vi "Run Process.vi"(0 "Time Left X":refnum<vi>, 1 "Completion X":refnum<vi>, 2 "Current Cycle Display X":refnum<vi>, 3 "ALD Sequence for Reactor X":refnum<vi>, 4 "Current Cycle Reactor X":refnum<vi>, 5 "Table Position Reactor X":refnum<vi>, 6 "Stop / Start Reactor X":refnum<vi>, 7 "System Idle X":refnum<vi>, 8 "Reactor Number (Base 0)":i32, 9 "Stop Program":refnum<vi>, 11 "System Queue":refnum<vi>, 12 "System Constants":T2, 13 "System JSON Queue":refnum<vi>, 14 "Reactor Selector":T1(ring), 15 "Current Locks":refnum<vi>, 17 "Current Valve State":refnum<vi>, 19 "Debug Mode":refnum<vi>, 20 "Wait Before Start (s) X":refnum<vi>, 21 "Timer Reactor X":refnum<vi>, 22 "Countdown X":refnum<vi>, 23 "Pressure (mTorr) X":refnum<vi>, 24 "Recorded Pressure X":refnum<vi>, 25 "Lock Reentrance Rate":refnum<vi>, 26 "Valve Close Delay":refnum<vi>) -> ()   [LabVIEW 2021]
uses:
  Valve State Machine.ctl
panel:
  out "Valves Per Shared Line":i32
  out "Number of Reactors":i32
  out "Valves Per Reactor":i32
  out "N2 Valves":i32[](array[numeric])
  out "Pump Valves":i32[](array[numeric])
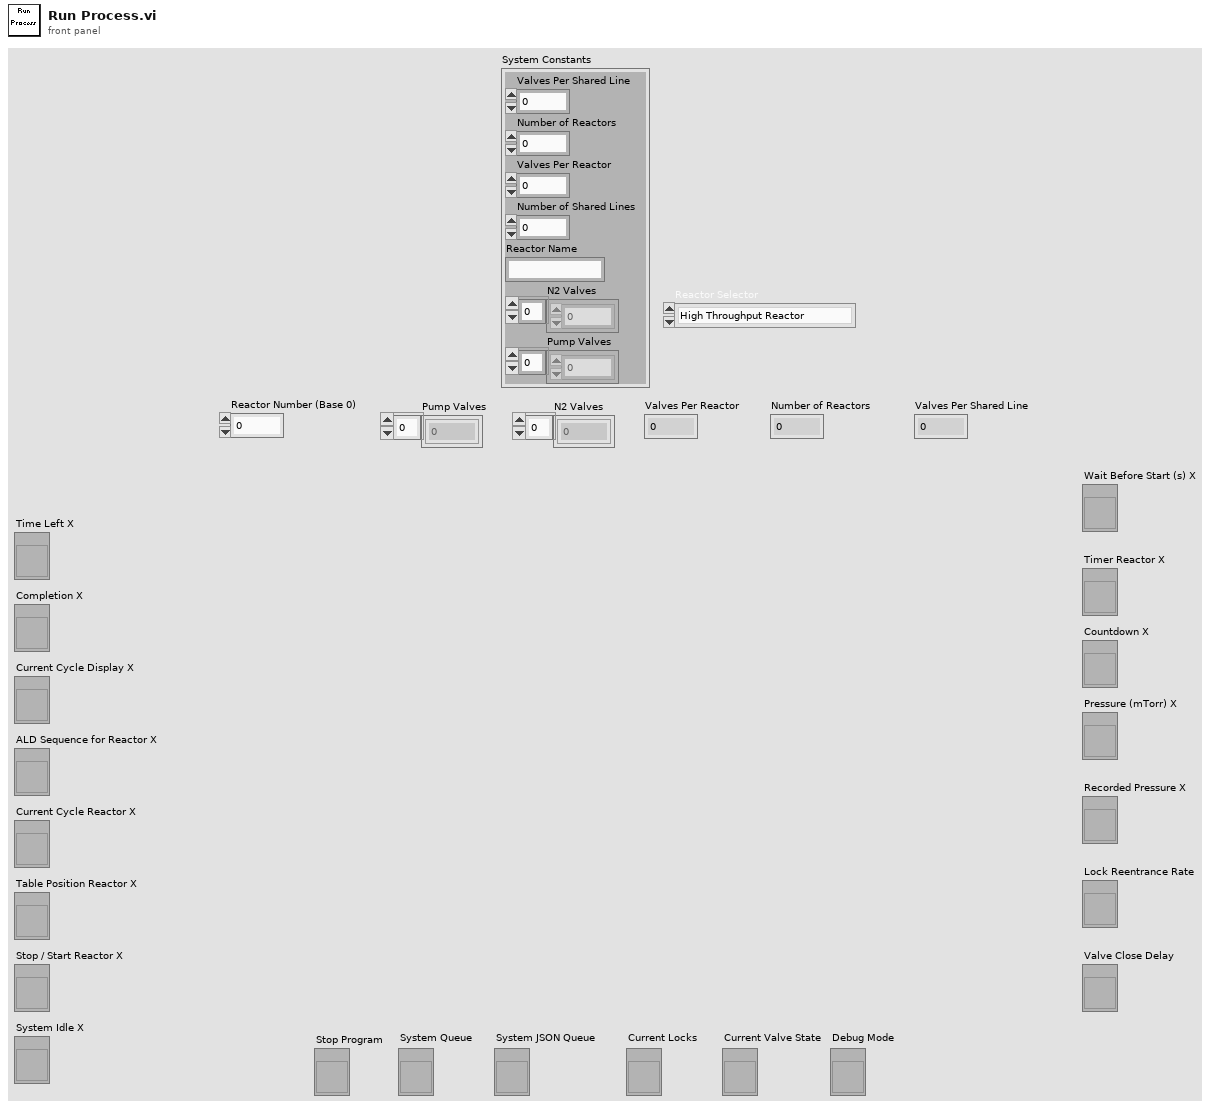
[diagram p1: front panel]
types:
  T1 = enum16{"High Throughput Reactor", "In Situ Reactor", "MLD Reactor"}
  T2 = cluster{"Valves Per Shared Line":i32, "Number of Reactors":i32, "Valves Per Reactor":i32, "Number of Shared Lines":i32, "Reactor Name":string, "N2 Valves":i32[], "Pump Valves":i32[]}
  T3 = typedef "Valve State Machine.ctl" = enum16{"0-Init Wait Before Start", "1-Wait Before Start", "2-Check Temp Request", "3-Claim Predose Pump Lock", "4-Init Predose Pump", "5-Wait Predose Pump", "6-Release Pump Lock", "7-Claim All Needed Locks", "8-Init N2Overlap", "9-Wait N2Overlap", "10-Init Pump Overlap", "11-Wait Pump Overlap", "12-Release Pump Lock", "13-Init Open Time", "14-Wait Open Time", "15-Release All Locks", "16-Init Hold", "17-Wait Hold", "18-Claim Pump Lock", "19-Init Pump Purge", "20-Wait Pump Purge", "21-Release Pump Lock", "22-Init Purge", "23-Wait Purge", "24-Check Purge Resume"}
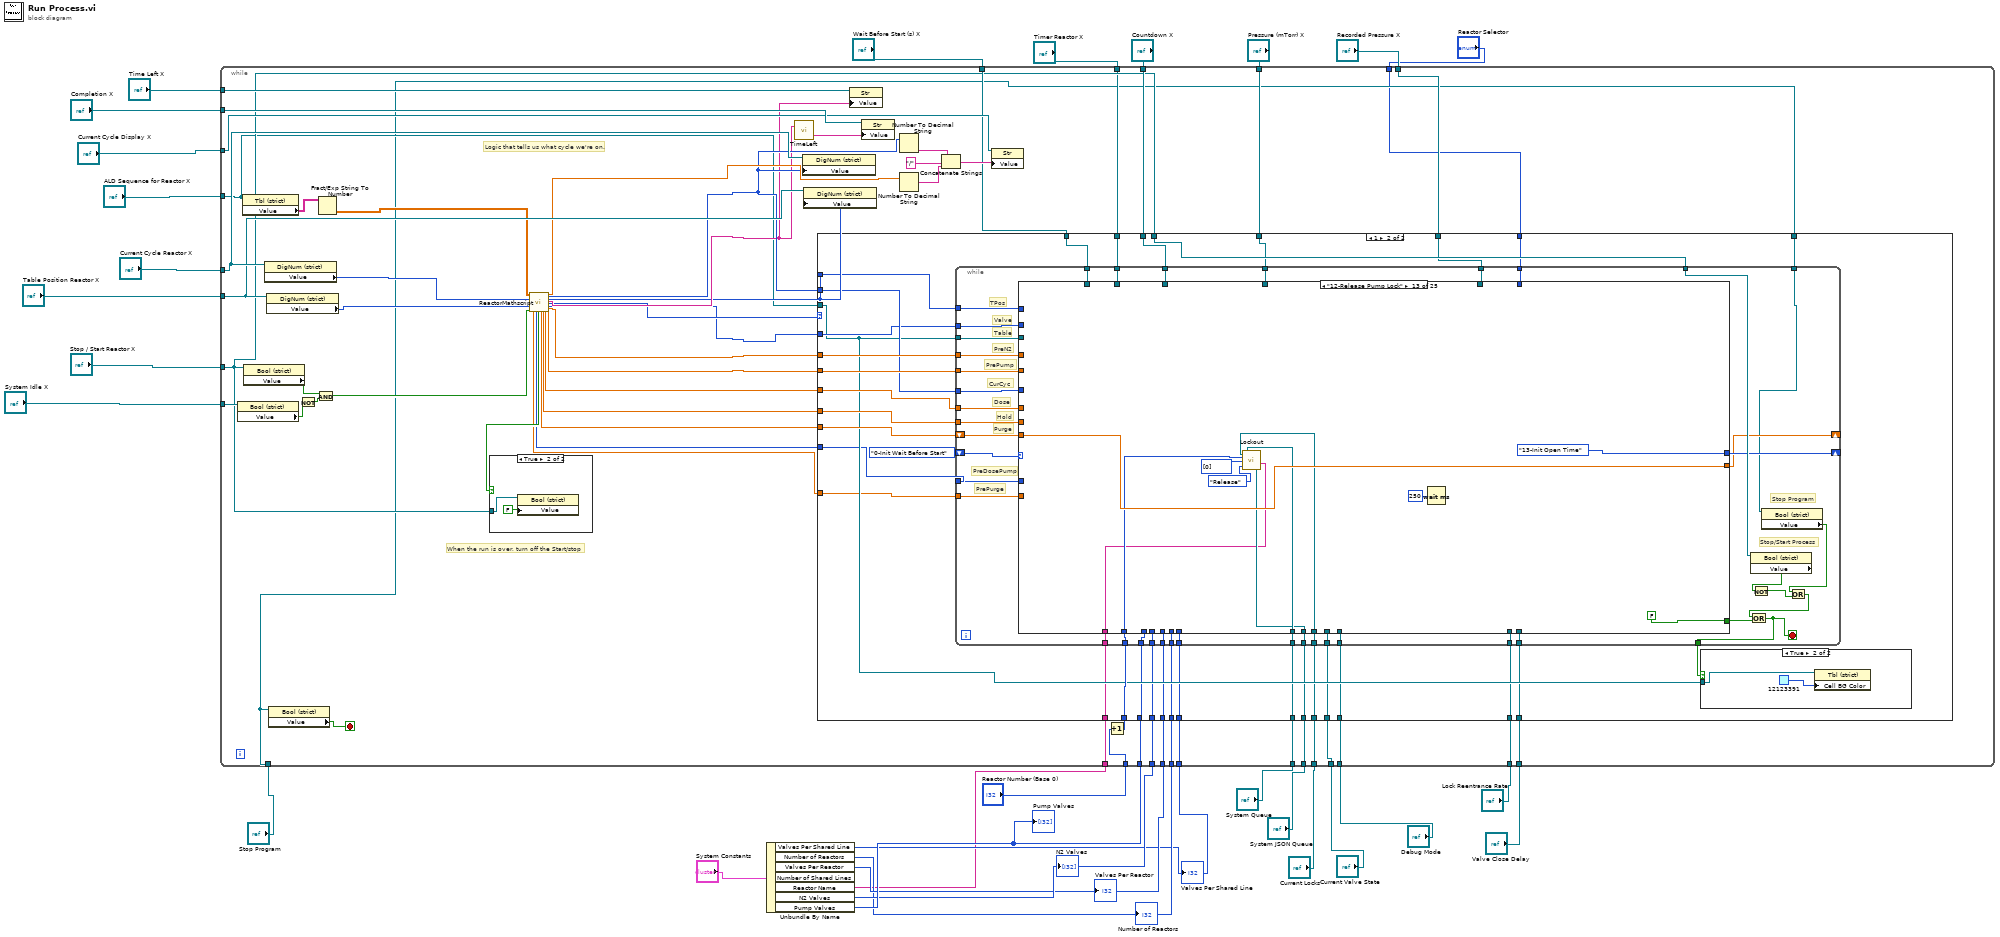
[diagram p0: block diagram]
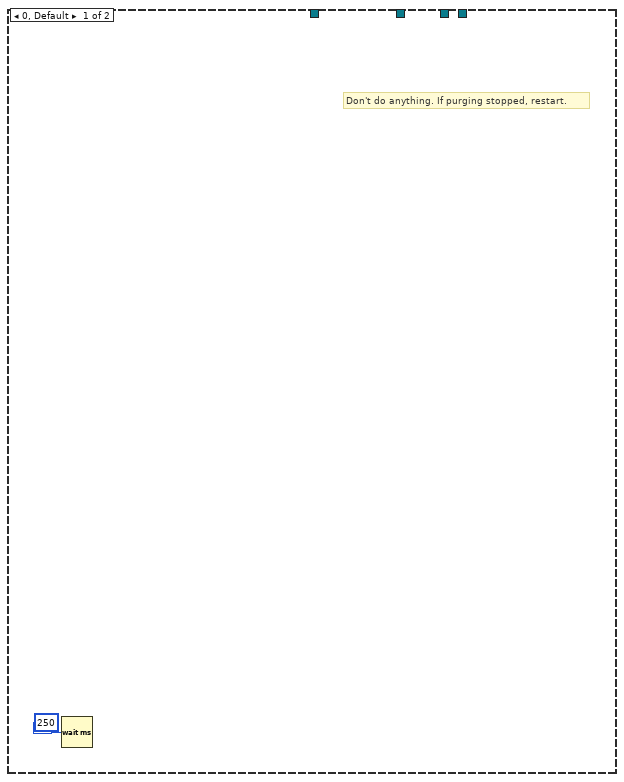
[diagram p3: hidden frame]
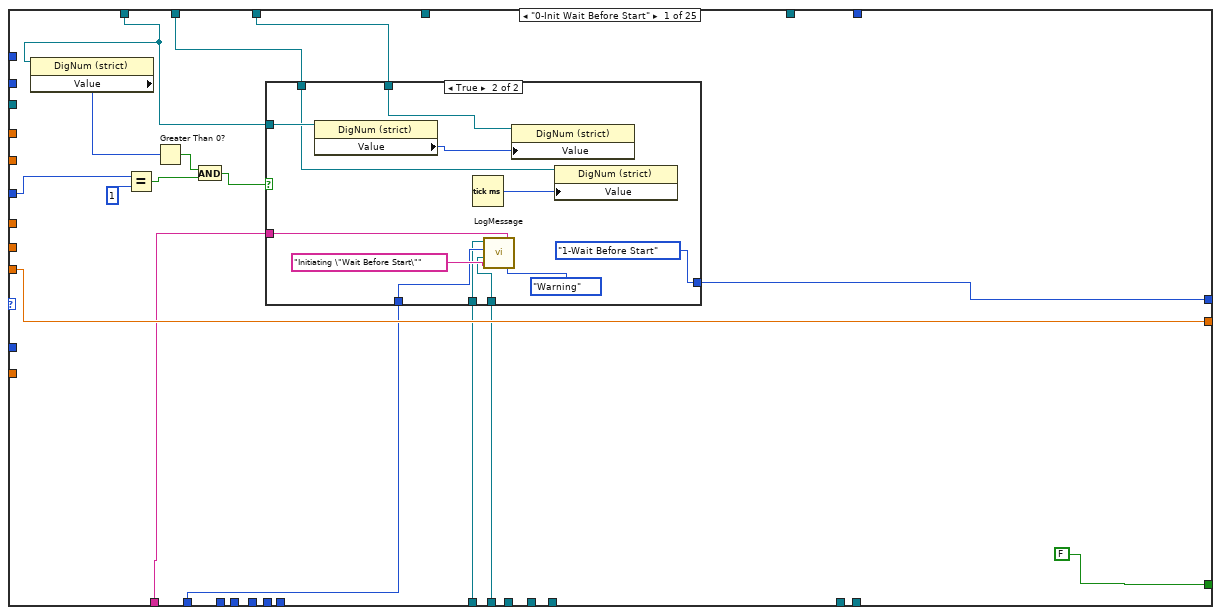
[diagram p5: hidden frame]
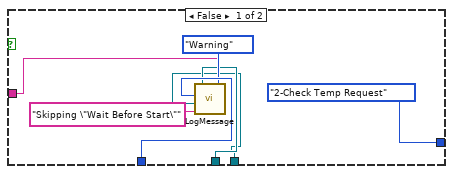
[diagram p6: hidden frame]
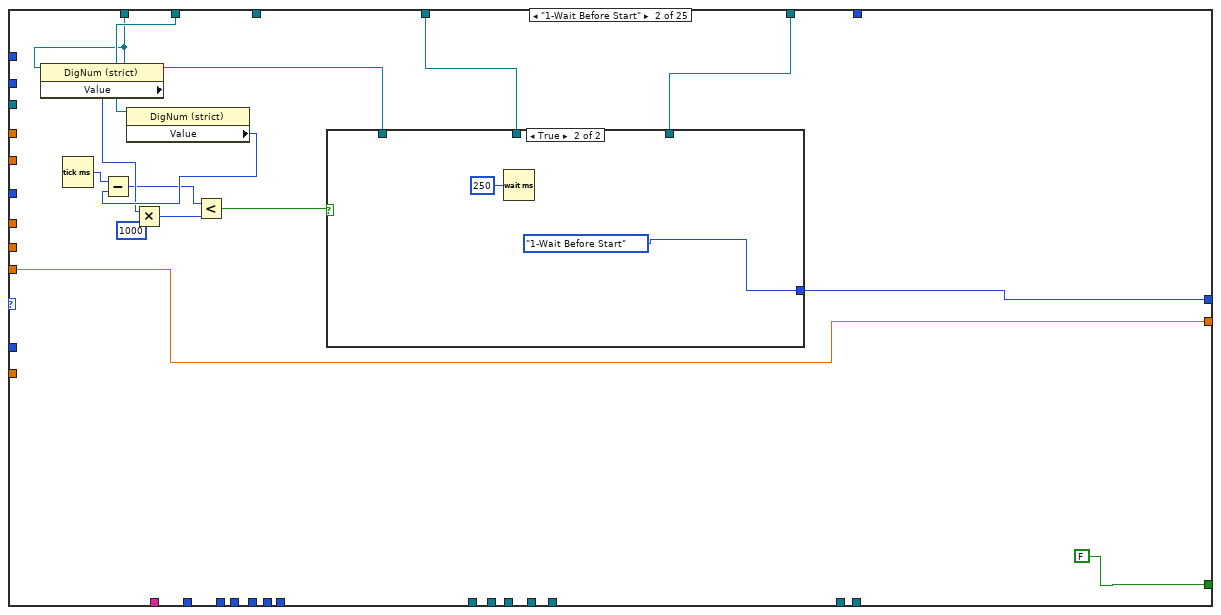
[diagram p7: hidden frame]
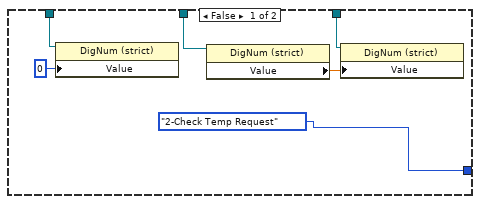
[diagram p8: hidden frame]
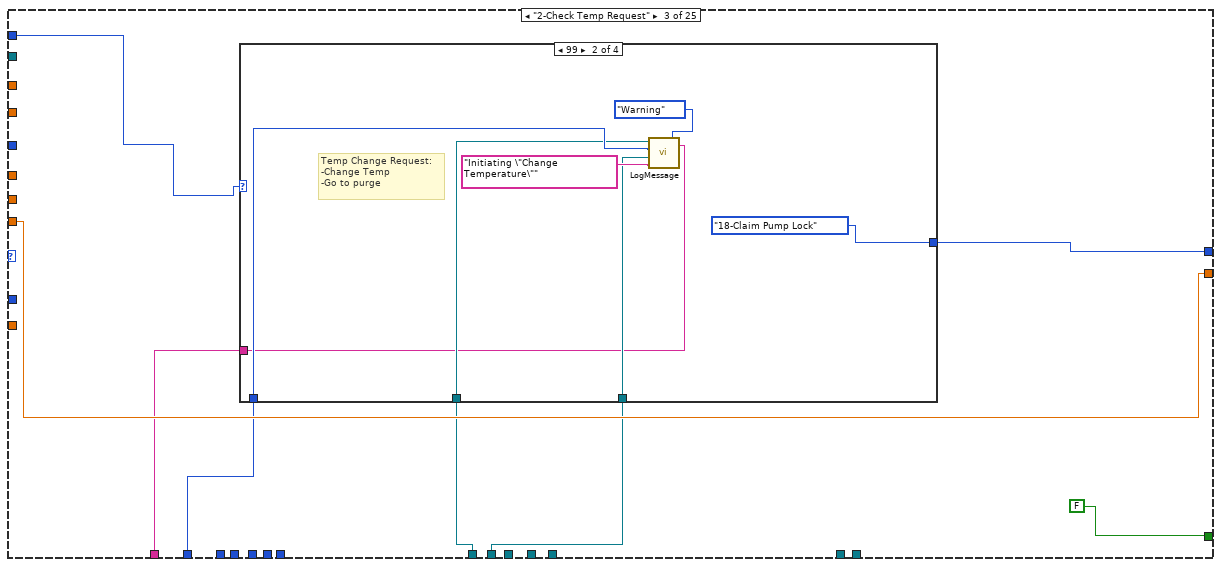
[diagram p9: hidden frame]
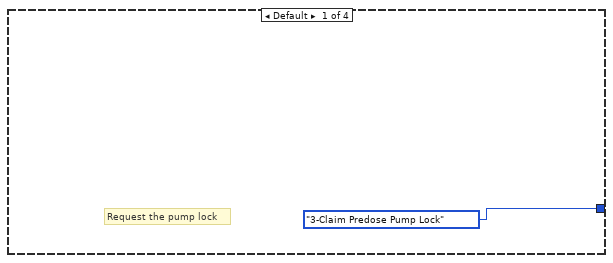
[diagram p10: hidden frame]
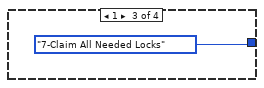
[diagram p11: hidden frame]
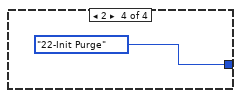
[diagram p12: hidden frame]
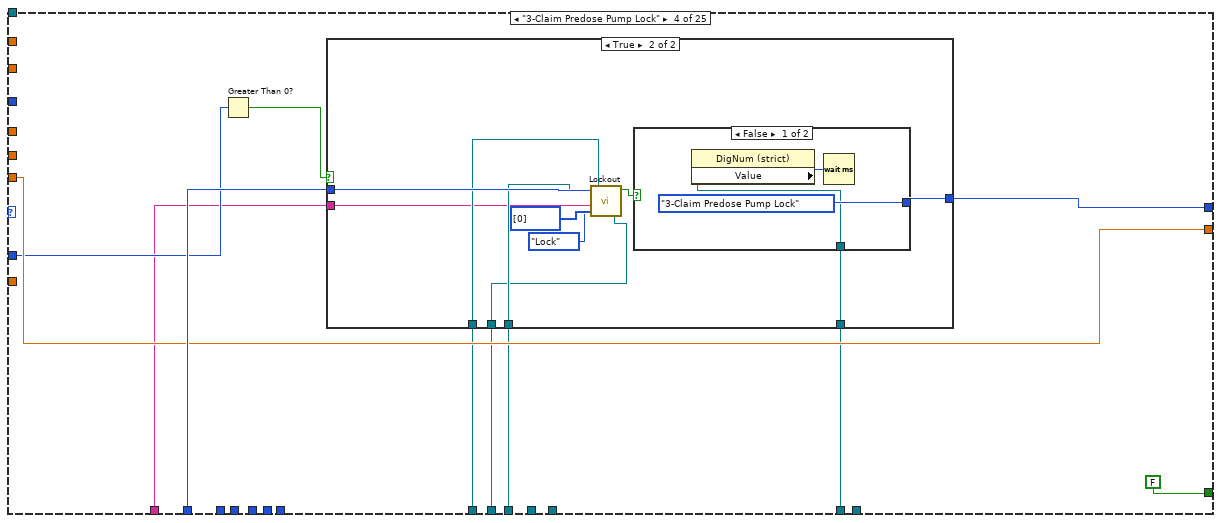
[diagram p13: hidden frame]
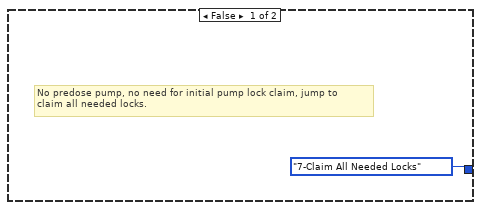
[diagram p14: hidden frame]
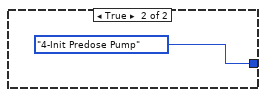
[diagram p15: hidden frame]
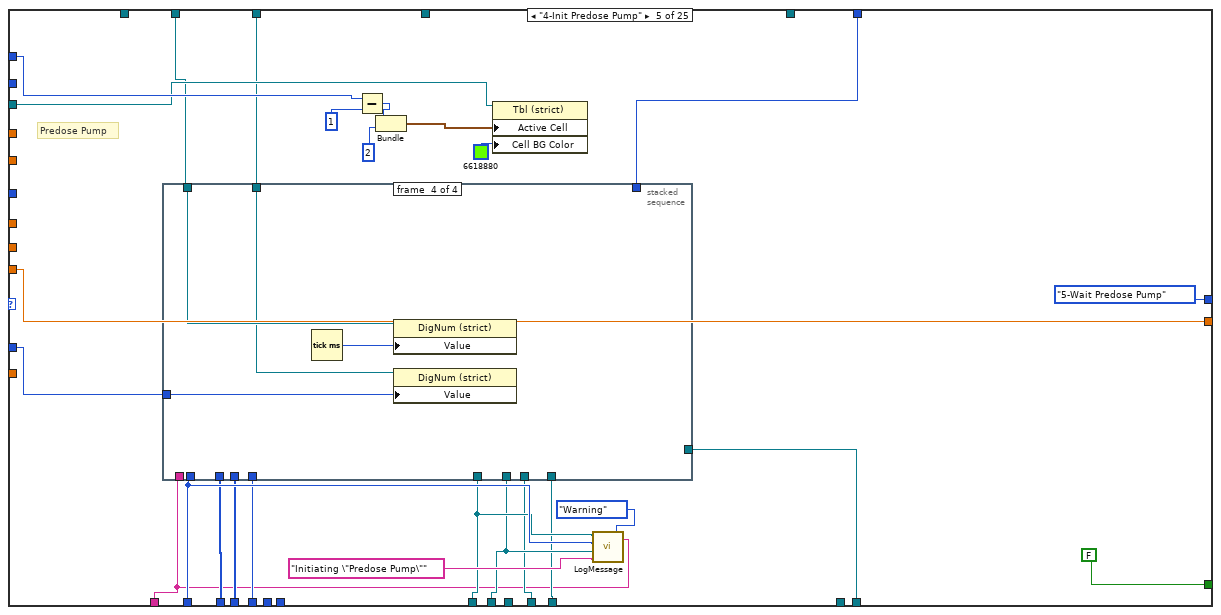
[diagram p16: hidden frame]
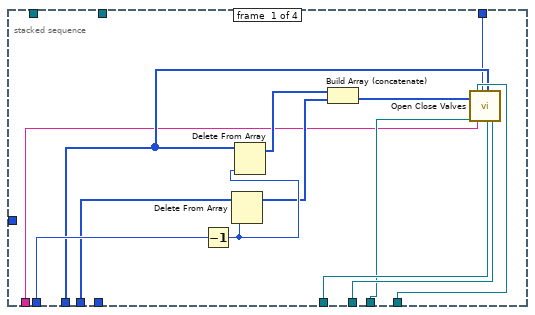
[diagram p17: hidden frame]
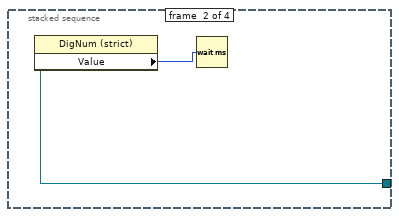
[diagram p18: hidden frame]
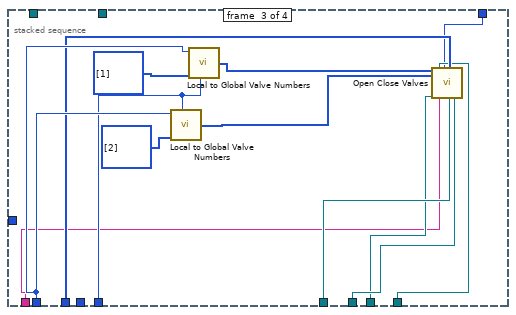
[diagram p19: hidden frame]
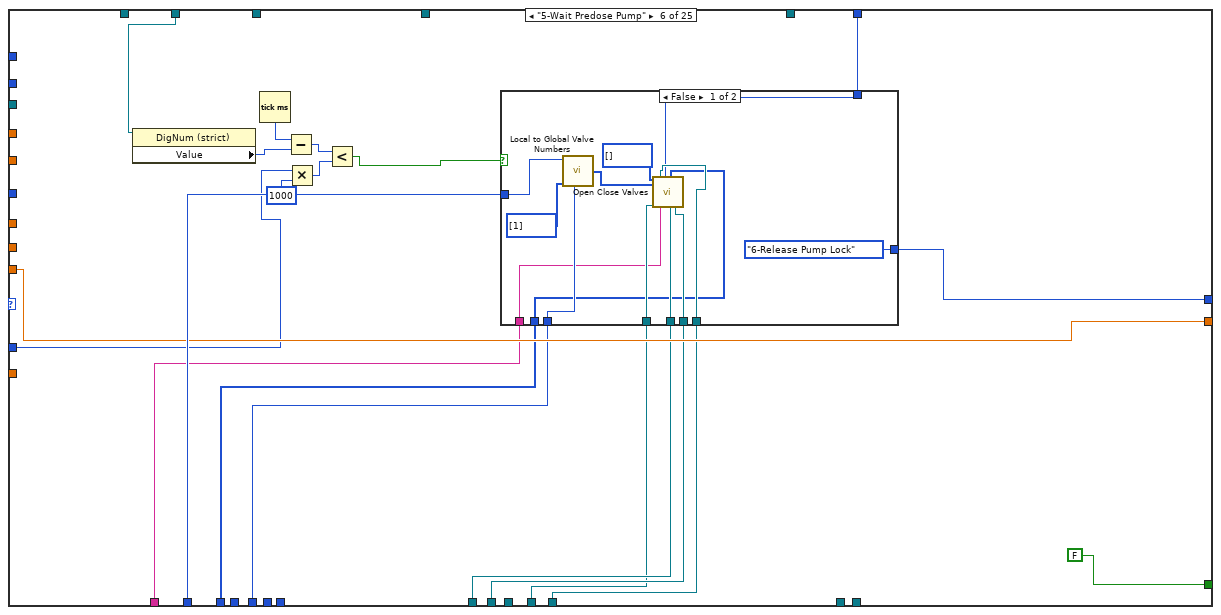
[diagram p20: hidden frame]
diagram:
  n1 = Unbundle By Name("System Constants") -> ("Valves Per Shared Line"=w3:i32, "Number of Reactors"=w4:i32, "Valves Per Reactor"=w5:i32, "Reactor Name"=w2:string, "N2 Valves"=w6:i32[], "Pump Valves"=w7:i32[])  [unwired: 1 out]
  "Pump Valves" <- w7
  "N2 Valves" <- w6
  "Valves Per Reactor" <- w5
  "Number of Reactors" <- w4
  "Valves Per Shared Line" <- w3
  n2 = while {
    tunnel: "Current Cycle Reactor X" -> [w85]
    tunnel: "Table Position Reactor X" -> [w81]
    tunnel: "ALD Sequence for Reactor X" -> [w49]
    tunnel: "System Idle X" -> [w88]
    tunnel: "Stop / Start Reactor X" -> [w60]
    tunnel: "Completion X" -> [w80]
    tunnel: "Time Left X" -> [w79]
    tunnel: "Current Cycle Display X" -> [w78]
    tunnel: "Wait Before Start (s) X" -> [w76]
    tunnel: "Countdown X" -> [w75]
    tunnel: "Pressure (mTorr) X" -> [w74]
    tunnel: "Recorded Pressure X" -> [w73]
    tunnel: "Reactor Number (Base 0)" -> [w72]
    tunnel: "Timer Reactor X" -> [w58]
    tunnel: "Stop Program" -> [w35]
    tunnel: "System Queue" -> [w45]
    tunnel: "System JSON Queue" -> [w44]
    tunnel: "Current Locks" -> [w43]
    tunnel: "Lock Reentrance Rate" -> [w42]
    tunnel: "Current Valve State" -> [w41]
    tunnel: "Debug Mode" -> [w40]
    tunnel: w7 -> [w39]
    tunnel: w6 -> [w38]
    tunnel: "Valve Close Delay" -> [w37]
    tunnel: w5 -> [w36]
    tunnel: w4 -> [w34]
    tunnel: w3 -> [w33]
    tunnel: w2 -> [w32]
    tunnel: "Reactor Selector" -> [w31]
    stop <- w46 stop-if-true
    # "When the run is over, turn off the Start/stop"
    # "Logic that tells us what cycle we're on."
    n3 = property class="Bool (strict)"(reference=w88) -> ("Value"=w86:bool)  [unwired: 1 in, 2 out]
    n4 = property class="Tbl (strict)"(reference=w49) -> ("Value"=w53:string[][])  [unwired: 1 in, 2 out]
    n5 = property class="Bool (strict)"(reference=w60) -> ("Value"=w87:bool)  [unwired: 1 in, 2 out]
    n6 = property class="DigNum (strict)"(reference=w85) -> ("Value"=w51:i32)  [unwired: 1 in, 2 out]
    n7 = property class="DigNum (strict)"(reference=w81) -> ("Value"=w52:i32)  [unwired: 1 in, 2 out]
    n8 = property class="Bool (strict)"(reference=w35) -> ("Value"=w46:bool)  [unwired: 1 in, 2 out]
    n9 = Not(x=w86) -> (.not. x?=w50:bool)
    n10 = And(x=w87, y=w50) -> (x .and. y?=w70:bool)
    n11 = Fract/Exp String To Number(string=w53) -> (number=w71:dbl[][])  [unwired: 3 in, 1 out]
    n12 = call "ReactorMathscript.vi"("T"=w71, "CurCycle"=w51, "TPos"=w52, "Run"=w70) -> ("PrePurge"=w47:dbl, "PreDosePump"=w48:i32, "StopRun"=w61:bool, "Purge"=w62:dbl, "Holds"=w63:dbl, "Dose"=w64:dbl, "TCyc"=w69:dbl, "CurCycle 2"=w68:i32, "TPos 2"=w56:i32, "TLeftStr"=w67:string, "Case"=w55:i32, "Valve"=w54:i32, "PreN2"=w66:dbl, "PrePump"=w65:dbl)  [unwired: 9 in, 1 out]
    n13 = case shown="True" w61 {
      tunnel: w60 -> [_ w90]
      frame False {
      }
      frame True {
        n14 = property class="Bool (strict)"(reference=w90, "Value"=FALSE) -> ()  [unwired: 1 in, 2 out]
      }
    }
    n15 = call "TimeLeft.vi"("Time Left"=w67) -> ("Completion"=w57:string)  [unwired: 2 in]
    n16 = property class="DigNum (strict)"(reference=w85, "Value"=w68) -> ()  [unwired: 1 in, 2 out]
    n17 = property class="DigNum (strict)"(reference=w81, "Value"=w56) -> ()  [unwired: 1 in, 2 out]
    n18 = property class="Str"(reference=w79, "Value"=w67) -> ()  [unwired: 1 in, 2 out]
    n19 = property class="Str"(reference=w80, "Value"=w57) -> ()  [unwired: 1 in, 2 out]
    n20 = Number To Decimal String(number=w68) -> (decimal integer string=w84:string)  [unwired: 1 in]
    n21 = Number To Decimal String(number=w69) -> (decimal integer string=w82:string)  [unwired: 1 in]
    n22 = Concatenate Strings(w84, "/", w82) -> (w77:string)
    n23 = property class="Str"(reference=w78, "Value"=w77) -> ()  [unwired: 1 in, 2 out]
    n24 = Increment(x=w72) -> (x+1=w59:i32)
    n25 = case shown="1" w55 {
      tunnel: w54 -> [_ w113]
      tunnel: w63 -> [_ w123]
      tunnel: w62 -> [_ w126]
      tunnel: w66 -> [_ w125]
      tunnel: w65 -> [_ w124]
      tunnel: w64 -> [_ w122]
      tunnel: w68 -> [_ w121]
      tunnel: w76 -> [_ w120]
      tunnel: w60 -> [_ w119]
      tunnel: w75 -> [_ w118]
      tunnel: w74 -> [_ w117]
      tunnel: w73 -> [_ w116]
      tunnel: w56 -> [_ w115]
      tunnel: w49 -> [_ w109]
      tunnel: w59 -> [_ w111]
      tunnel: w58 -> [_ w112]
      tunnel: w48 -> [_ w108]
      tunnel: w47 -> [_ w107]
      tunnel: w45 -> [_ w106]
      tunnel: w44 -> [_ w105]
      tunnel: w43 -> [_ w104]
      tunnel: w42 -> [_ w103]
      tunnel: w41 -> [_ w102]
      tunnel: w40 -> [_ w101]
      tunnel: w39 -> [_ w100]
      tunnel: w38 -> [_ w99]
      tunnel: w37 -> [_ w98]
      tunnel: w36 -> [_ w97]
      tunnel: w35 -> [_ w96]
      tunnel: w34 -> [_ w95]
      tunnel: w33 -> [_ w94]
      tunnel: w32 -> [_ w93]
      tunnel: w31 -> [_ w92]
      frame 0, Default {
        # "Don't do anything. If purging stopped, restart."
        n26 = Wait (ms)(milliseconds to wait=u32 250) -> ()  [unwired: 1 out]
      }
      frame 1 {
        n27 = while {
          shift-right: [w164] -> _
          shift-left: Valve_State_Machine."0-Init Wait Before Start" -> [w168]
          tunnel: w119 -> [w170]
          tunnel: w121 -> [w167]
          tunnel: w120 -> [w166]
          tunnel: w118 -> [w165]
          tunnel: w117 -> [w163]
          tunnel: w116 -> [w162]
          tunnel: w115 -> [w131]
          tunnel: w109 -> [w161]
          tunnel: w113 -> [w160]
          tunnel: w111 -> [w159]
          tunnel: w125 -> [w158]
          tunnel: w124 -> [w157]
          tunnel: w122 -> [w156]
          tunnel: w123 -> [w155]
          shift-right: [w153] -> _
          shift-left: w126 -> [w154]
          tunnel: w112 -> [w152]
          tunnel: [w150] -> w110
          tunnel: w108 -> [w149]
          tunnel: w107 -> [w148]
          tunnel: w106 -> [w147]
          tunnel: w105 -> [w146]
          tunnel: w104 -> [w145]
          tunnel: w103 -> [w144]
          tunnel: w102 -> [w143]
          tunnel: w101 -> [w142]
          tunnel: w100 -> [w141]
          tunnel: w99 -> [w140]
          tunnel: w98 -> [w139]
          tunnel: w97 -> [w138]
          tunnel: w96 -> [w136]
          tunnel: w95 -> [w133]
          tunnel: w94 -> [w132]
          tunnel: w93 -> [w130]
          tunnel: w92 -> [w129]
          stop <- w150 stop-if-true
          # "Stop/Start Process"
          # "Stop Program"
          # "PreDosePump"
          # "PrePurge"
          # "Purge"
          # "Hold"
          # "Dose"
          # "CurCyc"
          # "PrePump"
          # "PreN2"
          # "Table"
          # "Valve"
          # "TPos"
          n28 = case shown="\"12-Release Pump Lock\"" w168 {
            tunnel: [FALSE FALSE FALSE FALSE FALSE FALSE FALSE FALSE FALSE FALSE FALSE FALSE FALSE FALSE FALSE FALSE FALSE FALSE FALSE FALSE FALSE FALSE w1047 w1114 FALSE] -> w151
            tunnel: w167 -> [w176 _ _ _ _ _ _ _ _ _ _ _ _ _ _ _ _ _ _ _ _ _ _ _ _]
            tunnel: w166 -> [w180 w212 _ _ _ _ _ _ _ _ _ _ _ _ _ _ _ _ _ _ _ _ _ _ _]
            tunnel: w165 -> [w186 _ _ _ w283 _ _ _ w435 _ w606 _ _ w739 _ _ w862 _ _ w959 _ _ w1053 _ w1177]
            tunnel: [w182 w218 w234 w254 Valve_State_Machine."5-Wait Predose Pump" w349 Valve_State_Machine."7-Claim All Needed Locks" w397 w439 w543 w599 w688 Valve_State_Machine."13-Init Open Time" w734 w817 Valve_State_Machine."16-Init Hold" w857 w920 w935 w954 w1024 Valve_State_Machine."22-Init Purge" w1048 w1113 w1179] -> w164
            tunnel: w163 -> [_ w217 _ _ _ _ _ _ _ _ _ _ _ _ _ _ _ _ _ _ _ _ _ _ _]
            tunnel: w162 -> [_ w216 _ _ _ _ _ _ _ _ _ _ _ _ _ _ _ _ _ _ _ _ _ _ _]
            tunnel: w131 -> [_ _ _ _ w295 _ _ _ w434 _ w603 _ _ w738 _ _ w859 _ _ w956 _ _ w1051 _ _]
            tunnel: w161 -> [_ _ _ _ w294 _ _ _ w431 _ w604 _ _ w737 _ _ w860 _ _ w957 _ _ w1052 w1110 _]
            tunnel: w160 -> [_ _ w232 _ _ _ _ w375 w432 w532 w602 w676 _ w736 w805 _ w863 _ _ _ _ _ _ _ _]
            tunnel: w159 -> [w183 _ w231 w255 w285 w347 w371 w386 w433 w531 w601 w677 w715 w735 w806 w840 w858 _ w932 w955 _ w1033 w1050 w1111 _]
            tunnel: w158 -> [_ _ _ _ _ _ _ w393 w436 w533 _ _ _ _ _ _ _ _ _ _ _ _ _ _ _]
            tunnel: w157 -> [_ _ _ _ _ _ _ w389 _ _ w605 w679 _ _ _ _ _ _ _ _ _ _ _ _ _]
            tunnel: w156 -> [_ _ _ _ _ _ _ _ _ _ _ _ _ w740 w808 _ _ _ _ _ _ _ _ _ _]
            tunnel: w155 -> [_ _ _ _ _ _ _ _ _ _ _ _ _ _ _ _ w861 w910 _ _ _ _ _ _ _]
            tunnel: w154 -> [w184 w215 w233 w252 w288 w346 w372 w387 w430 w541 w598 w686 w717 w732 w815 w841 w855 w918 w933 w952 w1022 w1035 w1049 w1104 w1176]
            tunnel: [w184 w215 w233 w252 w288 w346 w372 w387 w430 w541 w598 w686 w717 w732 w815 w841 w855 w918 w933 w952 w1022 w1035 w1049 w1112 w1176] -> w153
            tunnel: w152 -> [w181 w214 _ _ w287 w339 _ _ w429 w534 w597 w678 _ w731 w807 _ w854 w911 _ w951 w1015 _ w1046 w1102 _]
            tunnel: w149 -> [_ _ _ w251 w282 w338 _ _ _ _ _ _ _ _ _ _ _ _ _ _ _ _ _ _ _]
            tunnel: w148 -> [_ _ _ _ _ _ _ _ _ _ _ _ _ _ _ _ _ _ _ w950 w1014 _ _ _ _]
            tunnel: w147 -> [w173 _ w230 w249 w281 w337 w367 w381 w426 w525 w591 w673 w712 w728 w798 w836 w848 _ w928 w945 _ w1030 w1044 w1099 w1169]
            tunnel: w146 -> [w172 _ w229 w248 w280 w336 w368 w382 w425 w524 w590 w672 w711 w727 w797 w835 w847 _ w927 w944 _ w1029 w1045 w1098 w1170]
            tunnel: w145 -> [_ _ _ w250 _ _ w366 w380 _ _ _ _ w710 _ _ w837 _ _ w926 _ _ w1031 _ _ w1171]
            tunnel: w144 -> [_ _ _ w247 _ _ _ w379 _ _ _ _ _ _ _ _ _ _ w925 _ _ _ _ _ w1168]
            tunnel: w143 -> [_ _ _ _ w279 w335 _ _ w422 w527 w589 w675 _ w729 w800 _ w849 _ _ w946 _ _ w1041 w1101 _]
            tunnel: w142 -> [_ _ _ _ w278 w334 _ _ w423 w526 w588 w674 _ w730 w799 _ w846 _ _ w943 _ _ w1042 _ _]
            tunnel: w141 -> [_ _ _ _ w277 w332 _ _ w421 w523 w593 w668 _ w722 w801 _ w850 _ _ w949 _ _ w1043 _ _]
            tunnel: w140 -> [_ _ _ _ w276 _ _ _ w420 _ w592 _ _ _ _ _ _ _ _ w948 _ _ _ _ _]
            tunnel: w139 -> [_ _ _ _ w275 _ _ _ w419 _ w587 _ _ w726 _ _ _ _ _ w942 _ _ _ _ _]
            tunnel: w138 -> [_ _ _ _ w274 w333 _ _ w427 w529 w595 w671 _ w724 w804 _ w853 _ _ w947 _ _ w1040 w1100 _]
            tunnel: w133 -> [_ _ _ _ _ _ _ _ w428 w530 w594 w670 _ w725 w803 _ w852 _ _ _ _ _ _ _ _]
            tunnel: w132 -> [_ _ _ _ _ _ _ _ w424 w528 w596 w669 _ w723 w802 _ w851 _ _ _ _ _ _ _ _]
            tunnel: w130 -> [w171 _ w228 w246 w273 w331 w365 w378 w418 w522 w586 w667 w709 w721 w796 w834 w845 _ w924 w941 _ w1028 w1039 w1097 w1167]
            tunnel: w129 -> [_ _ _ _ w272 w330 _ _ w417 w521 w585 w666 _ w720 w795 _ w844 _ _ w940 _ _ w1038 _ _]
            frame "0-Init Wait Before Start" {
              n29 = property class="DigNum (strict)"(reference=w180) -> ("Value"=w179:i32)  [unwired: 1 in, 2 out]
              n30 = Equal?(x=w176, y=1) -> (x = y?=w174:bool)
              n31 = Greater Than 0?(x=w179) -> (x > 0?=w178:bool)
              n32 = And(x=w178, y=w174) -> (x .and. y?=w177:bool)
              n33 = case shown="True" w177 {
                tunnel: w180 -> [_ w205]
                tunnel: w186 -> [_ w204]
                tunnel: w183 -> [w191 w198]
                tunnel: [Valve_State_Machine."2-Check Temp Request" Valve_State_Machine."1-Wait Before Start"] -> w182
                tunnel: w181 -> [_ w201]
                tunnel: w173 -> [w189 w196]
                tunnel: w172 -> [w188 w195]
                tunnel: w171 -> [w187 w194]
                frame False {
                  n34 = call "LogMessage.vi"("Type"=enum16{"Locks", "Warning"}."Warning", "Reactor Name"=w187, "Log Entry"="Skipping \"Wait Before Start\"", "System JSON Queue"=w188, "ID Number"=w191, "System Queue"=w189) -> ()
                }
                frame True {
                  n35 = property class="DigNum (strict)"(reference=w205) -> ("Value"=w203:i32)  [unwired: 1 in, 2 out]
                  n36 = Tick Count (ms)() -> (millisecond timer value=w200:u32)
                  n37 = call "LogMessage.vi"("Type"=enum16{"Locks", "Warning"}."Warning", "Reactor Name"=w194, "Log Entry"="Initiating \"Wait Before Start\"", "System JSON Queue"=w195, "ID Number"=w198, "System Queue"=w196) -> ()
                  n38 = property class="DigNum (strict)"(reference=w204, "Value"=w203) -> ()  [unwired: 1 in, 2 out]
                  n39 = property class="DigNum (strict)"(reference=w201, "Value"=w200) -> ()  [unwired: 1 in, 2 out]
                }
              }
            }
            frame "1-Wait Before Start" {
              n40 = property class="DigNum (strict)"(reference=w212) -> ("Value"=w209:i32)  [unwired: 1 in, 2 out]
              n41 = Tick Count (ms)() -> (millisecond timer value=w213:u32)
              n42 = property class="DigNum (strict)"(reference=w214) -> ("Value"=w211:i32)  [unwired: 1 in, 2 out]
              n43 = Subtract(x=w213, y=w211) -> (x-y=w207:u32)
              n44 = Multiply(x=w209, y=1000) -> (x*y=w206:i32)
              n45 = Less?(x=w207, y=w206) -> (x < y?=w210:bool)
              n46 = case shown="True" w210 {
                tunnel: [Valve_State_Machine."2-Check Temp Request" Valve_State_Machine."1-Wait Before Start"] -> w218
                tunnel: w212 -> [w225 _]
                tunnel: w217 -> [w223 _]
                tunnel: w216 -> [w222 _]
                frame False {
                  n47 = property class="DigNum (strict)"(reference=w225, "Value"=0) -> ()  [unwired: 1 in, 2 out]
                  n48 = property class="DigNum (strict)"(reference=w223) -> ("Value"=w221:dbl)  [unwired: 1 in, 2 out]
                  n49 = property class="DigNum (strict)"(reference=w222, "Value"=w221) -> ()  [unwired: 1 in, 2 out]
                }
                frame True {
                  n50 = Wait (ms)(milliseconds to wait=u32 250 ("millisecond multiple")) -> ()  [unwired: 1 out]
                }
              }
            }
            frame "2-Check Temp Request" {
              n51 = case shown="99" w232 {
                tunnel: [Valve_State_Machine."3-Claim Predose Pump Lock" Valve_State_Machine."18-Claim Pump Lock" Valve_State_Machine."7-Claim All Needed Locks" Valve_State_Machine."22-Init Purge"] -> w234
                tunnel: w231 -> [_ w241 _ _]
                tunnel: w230 -> [_ w239 _ _]
                tunnel: w229 -> [_ w238 _ _]
                tunnel: w228 -> [_ w237 _ _]
                frame Default {
                  # "Request the pump lock"
                }
                frame 99 {
                  # "Temp Change Request:\n-Change Temp\n-Go to purge"
                  n52 = call "LogMessage.vi"("Type"=enum16{"Locks", "Warning"}."Warning", "Reactor Name"=w237, "Log Entry"="Initiating \"Change Temperature\"", "System JSON Queue"=w238, "ID Number"=w241, "System Queue"=w239) -> ()
                }
                frame 1 {
                }
                frame 2 {
                }
              }
            }
            frame "3-Claim Predose Pump Lock" {
              n53 = Greater Than 0?(x=w251) -> (x > 0?=w256:bool)
              n54 = case shown="True" w256 {
                tunnel: w255 -> [_ w266]
                tunnel: [Valve_State_Machine."7-Claim All Needed Locks" w267] -> w254
                tunnel: w250 -> [_ w262]
                tunnel: w249 -> [_ w261]
                tunnel: w248 -> [_ w260]
                tunnel: w247 -> [_ w259]
                tunnel: w246 -> [_ w258]
                frame False {
                  # "No predose pump, no need for initial pump lock claim, jump to\nclaim all needed locks."
                }
                frame True {
                  n55 = call "Lockout.vi"("Locks"=w262, "ID"=w266, "Queue System"=w261, "Request Type"=enum16{"Lock", "Release", "Check"}."Lock", "Request Array"=i32[] [0], "Reactor Name"=w258, "JSON Queue"=w260) -> ("Response"=w263:bool)  [unwired: 1 out]
                  n56 = case shown="False" w263 {
                    tunnel: [Valve_State_Machine."3-Claim Predose Pump Lock" Valve_State_Machine."4-Init Predose Pump"] -> w267
                    tunnel: w259 -> [w268 _]
                    frame False {
                      n57 = property class="DigNum (strict)"(reference=w268) -> ("Value"=w269:i32)  [unwired: 1 in, 2 out]
                      n58 = Wait (ms)(milliseconds to wait=w269) -> ()  [unwired: 1 out]
                    }
                    frame True {
                    }
                  }
                }
              }
            }
            frame "4-Init Predose Pump" {
              # "Predose Pump"
              n59 = stacked-sequence {
                tunnel: w285 -> [w307 _ w323 _]
                tunnel: w287 -> [_ _ _ w328]
                tunnel: w283 -> [_ _ _ w327]
                tunnel: w282 -> [_ _ _ w326]
                tunnel: w281 -> [w305 _ w317 _]
                tunnel: w280 -> [w304 _ w316 _]
                tunnel: w279 -> [w303 _ w315 _]
                tunnel: w278 -> [w302 _ w318 _]
                tunnel: w277 -> [w301 _ w319 _]
                tunnel: w276 -> [w300 _ _ _]
                tunnel: w275 -> [_ w311 _ _]
                tunnel: w274 -> [_ _ w320 _]
                tunnel: w273 -> [w299 _ w314 _]
                tunnel: w272 -> [w298 _ w313 _]
                frame #0 {
                  n60 = Decrement(x=w307) -> (x-1=w310:i32)
                  n61 = Delete From Array(array=w300, index=w310) -> (array with subset deleted=w308:i32[])  [unwired: 1 in, 1 out]
                  n62 = Delete From Array(array=w301, index=w310) -> (array with subset deleted=w309:i32[])  [unwired: 1 in, 1 out]
                  n63 = Build Array (concatenate)(w309, w308) -> (w306:i32[])
                  n64 = call "Open Close Valves.vi"("Valves to Close"=w306, "Current Valve State"=w303, "Debug Mode"=w302, "Reactor Name"=w299, "Reactor Selector"=w298, "Pump Valves"=w301, "System Queue"=w305, "JSON Queue"=w304) -> ()  [unwired: 12 in]
                }
                frame #1 {
                  n65 = property class="DigNum (strict)"(reference=w311) -> ("Value"=w312:i32)  [unwired: 1 in, 2 out]
                  n66 = Wait (ms)(milliseconds to wait=w312) -> ()  [unwired: 1 out]
                }
                frame #2 {
                  n67 = call "Local to Global Valve Numbers.vi"("Reactor ID #"=w323, "List of Local Valves"=i32[] [2], "Valves Per Reactor"=w320) -> ("List of Global Valves"=w321:i32[])  [unwired: 2 in]
                  n68 = call "Local to Global Valve Numbers.vi"("Reactor ID #"=w323, "List of Local Valves"=i32[] [1] ("Valves to Open"), "Valves Per Reactor"=w320) -> ("List of Global Valves"=w322:i32[])  [unwired: 2 in]
                  n69 = call "Open Close Valves.vi"("Valves to Open"=w322, "Valves to Close"=w321, "Current Valve State"=w315, "Debug Mode"=w318, "Reactor Name"=w314, "Reactor Selector"=w313, "Pump Valves"=w319, "System Queue"=w317, "JSON Queue"=w316) -> ()  [unwired: 11 in]
                }
                frame #3 {
                  n70 = Tick Count (ms)() -> (millisecond timer value=w329:u32)
                  n71 = property class="DigNum (strict)"(reference=w328, "Value"=w329) -> ()  [unwired: 1 in, 2 out]
                  n72 = property class="DigNum (strict)"(reference=w327, "Value"=w326) -> ()  [unwired: 1 in, 2 out]
                }
              }
              n73 = Subtract(x=w295, y=1) -> (x-y=w293:i32)
              n74 = Bundle(w293, 2) -> (w292:cluster{i32, i32})  [unwired: 1 in]
              n75 = property class="Tbl (strict)"(reference=w294, "Active Cell"=w292, "Cell BG Color"=u32 6618880) -> ()  [unwired: 1 in, 2 out]
              n76 = call "LogMessage.vi"("Type"=enum16{"Locks", "Warning"}."Warning", "Reactor Name"=w273, "Log Entry"="Initiating \"Predose Pump\"", "System JSON Queue"=w280, "ID Number"=w285, "System Queue"=w281) -> ()
            }
            frame "5-Wait Predose Pump" {
              n77 = property class="DigNum (strict)"(reference=w339) -> ("Value"=w342:i32)  [unwired: 1 in, 2 out]
              n78 = Tick Count (ms)() -> (millisecond timer value=w341:u32)
              n79 = Subtract(x=w341, y=w342) -> (x-y=w343:u32)
              n80 = Multiply(x=w338, y=1000) -> (x*y=w344:i32)
              n81 = Less?(x=w343, y=w344) -> (x < y?=w340:bool)
              n82 = case shown="False" w340 {
                tunnel: [Valve_State_Machine."6-Release Pump Lock" Valve_State_Machine."5-Wait Predose Pump"] -> w349
                tunnel: w347 -> [w361 _]
                tunnel: w337 -> [w357 _]
                tunnel: w336 -> [w356 _]
                tunnel: w335 -> [w355 _]
                tunnel: w334 -> [w354 _]
                tunnel: w333 -> [w353 _]
                tunnel: w332 -> [w352 _]
                tunnel: w331 -> [w351 _]
                tunnel: w330 -> [w350 _]
                frame False {
                  n83 = call "Local to Global Valve Numbers.vi"("Reactor ID #"=w361, "List of Local Valves"=i32[] [1], "Valves Per Reactor"=w353) -> ("List of Global Valves"=w359:i32[])  [unwired: 2 in]
                  n84 = call "Open Close Valves.vi"("Valves to Open"=i32[] [], "Valves to Close"=w359, "Current Valve State"=w355, "Debug Mode"=w354, "Reactor Name"=w351, "Reactor Selector"=w350, "Pump Valves"=w352, "System Queue"=w357, "JSON Queue"=w356) -> ()  [unwired: 11 in]
                }
                frame True {
                  n85 = Wait (ms)(milliseconds to wait=u32 250 ("millisecond multiple")) -> ()  [unwired: 1 out]
                }
              }
            }
            frame "6-Release Pump Lock" {
              n86 = call "Lockout.vi"("Locks"=w366, "ID"=w371, "Queue System"=w367, "Request Type"=enum16{"Lock", "Release", "Check"}."Release", "Request Array"=i32[] [0], "Reactor Name"=w365, "JSON Queue"=w368) -> ()  [unwired: 2 out]
            }
            frame "7-Claim All Needed Locks" {
              n87 = Not Equal?(x=w375, y=2) -> (x != y?=w394:bool)
              n88 = Greater Than 0?(x=w393) -> (x > 0?=w392:bool)
              n89 = Greater Than 0?(x=w389) -> (x > 0?=w390:bool)
              n90 = And(x=w394, y=w392) -> (x .and. y?=w391:bool)
              n91 = Or(x=w391, y=w390) -> (x .or. y?=w388:bool)
              n92 = Greater?(x=w375, y=50) -> (0:w377:bool)
              n93 = case shown="True" w388 {
                tunnel: [i32[] [] i32[] [0]] -> w398
                frame False {
                  # "Purge only"
                }
                frame True {
                }
              }
              n94 = case shown="True" w377 {
                tunnel: w398 -> [w409 w413]
                tunnel: [w409 w412] -> w385
                tunnel: w375 -> [_ w411]
                frame False {
                }
                frame True {
                  n95 = Quotient & Remainder(x=w411, y=10) -> (floor(x/y)=w416:i32)  [unwired: 1 out]
                  n96 = Subtract(x=w416, y=4) -> (x-y=w410:i32)
                  n97 = Build Array (concatenate)(w413, w410) -> (w412:i32[])
                }
              }
              n98 = call "Lockout.vi"("Locks"=w380, "ID"=w386, "Queue System"=w381, "Request Type"=enum16{"Lock", "Release", "Check"}."Lock", "Request Array"=w385, "Reactor Name"=w378, "JSON Queue"=w382) -> ("Response"=w383:bool)  [unwired: 1 out]
              n99 = case shown="False" w383 {
                tunnel: [Valve_State_Machine."6-Release Pump Lock" w404] -> w397
                tunnel: w375 -> [_ w405]
                tunnel: w379 -> [w401 _]
                frame False {
                  n100 = property class="DigNum (strict)"(reference=w401) -> ("Value"=w402:i32)  [unwired: 1 in, 2 out]
                  n101 = Wait (ms)(milliseconds to wait=w402) -> ()  [unwired: 1 out]
                }
                frame True {
                  n102 = case shown="1" w405 {
                    tunnel: [Valve_State_Machine."8-Init N2Overlap" Valve_State_Machine."10-Init Pump Overlap" Valve_State_Machine."22-Init Purge"] -> w404
                    frame Default {
                    }
                    frame 1 {
                    }
                    frame 2 {
                    }
                  }
                }
              }
            }
            frame "8-Init N2Overlap" {
              # "Pump Open\nNitrogen Open"
              n103 = Greater Than 0?(x=w436) -> (x > 0?=w437:bool)
              n104 = case shown="True" w437 {
                tunnel: [Valve_State_Machine."10-Init Pump Overlap" Valve_State_Machine."9-Wait N2Overlap"] -> w439
                tunnel: w436 -> [_ w456]
                tunnel: w435 -> [_ w457]
                tunnel: w434 -> [_ w471]
                tunnel: w433 -> [_ w459]
                tunnel: w432 -> [_ w444]
                tunnel: w431 -> [_ w467]
                tunnel: w429 -> [_ w463]
                tunnel: w428 -> [_ w455]
                tunnel: w427 -> [_ w454]
                tunnel: w426 -> [_ w452]
                tunnel: w425 -> [_ w451]
                tunnel: w424 -> [_ w453]
                tunnel: w423 -> [_ w450]
                tunnel: w422 -> [_ w449]
                tunnel: w421 -> [_ w448]
                tunnel: w420 -> [_ w447]
                tunnel: w419 -> [_ w446]
                tunnel: w418 -> [_ w442]
                tunnel: w417 -> [_ w441]
                frame False {
                }
                frame True {
                  n105 = Greater?(x=w444, y=50) -> (0:w445:bool)
                  n106 = case shown="True" w445 {
                    tunnel: [w515 w518] -> w462
                    tunnel: w459 -> [w511 w519]
                    tunnel: w455 -> [w509 _]
                    tunnel: w454 -> [w508 w517]
                    tunnel: w453 -> [w503 _]
                    tunnel: w444 -> [w507 _]
                    frame True {
                      n107 = Quotient & Remainder(x=w507, y=10) -> (floor(x/y)=w506:i32)  [unwired: 1 out]
                      n108 = Subtract(x=w506, y=5) -> (x-y=w504:i32)
                      n109 = Multiply(x=w504, y=w503) -> (x*y=w502:i32)
                      n110 = call "Local to Global Valve Numbers.vi"("Reactor ID #"=w511, "List of Local Valves"=i32[] [1], "Valves Per Reactor"=w508) -> ("List of Global Valves"=w510:i32[])  [unwired: 2 in]
                      n111 = Multiply(x=w508, y=w509) -> (x*y=w514:i32)
                      n112 = Add(x=w514, y=w502) -> (x+y=w513:i32)
                      n113 = Increment(x=w513) -> (x+1=w516:i32)
                      n114 = Build Array (concatenate)(w510, w516) -> (w515:i32[])
                    }
                    frame False {
                      n115 = call "Local to Global Valve Numbers.vi"("Reactor ID #"=w519, "List of Local Valves"=i32[] [1, 2], "Valves Per Reactor"=w517) -> ("List of Global Valves"=w518:i32[])  [unwired: 2 in]
                    }
                  }
                  n116 = call "Convert Recipe Valve to Valve List.vi"("Valves on Shared Lines"=w453, "Valves Per Reactor"=w454, "Number of Reactors"=w455, "Reactor ID#"=w459, "Valve Number"=w444) -> ("Valve List"=w466:i32[])  [unwired: 10 in]
                  n117 = Build Array (concatenate)(w466, w462) -> (w465:i32[])
                  n118 = Subtract(x=w471, y=1) -> (x-y=w474:i32)
                  n119 = Bundle(w474, 3) -> (w470:cluster{i32, i32})  [unwired: 1 in]
                  n120 = Decrement(x=w459) -> (x-1=w461:i32)
                  n121 = property class="Tbl (strict)"(reference=w467, "Cell BG Color"=u32 12123391, "Active Cell"=w470, "Cell BG Color"=u32 16318208) -> ()  [unwired: 1 in, 2 out]
                  n122 = stacked-sequence {
                    tunnel: w465 -> [_ _ w496 _]
                    tunnel: w463 -> [_ _ _ w499]
                    tunnel: w461 -> [w483 _ _ _]
                    tunnel: w457 -> [_ _ _ w498]
                    tunnel: w456 -> [_ _ _ w497]
                    tunnel: w452 -> [w482 _ w493 _]
                    tunnel: w451 -> [w481 _ w492 _]
                    tunnel: w450 -> [w480 _ w495 _]
                    tunnel: w449 -> [w479 _ w494 _]
                    tunnel: w448 -> [w478 _ w491 _]
                    tunnel: w447 -> [w477 _ _ _]
                    tunnel: w446 -> [_ w487 _ _]
                    tunnel: w442 -> [w476 _ w490 _]
                    tunnel: w441 -> [w475 _ w489 _]
                    frame #0 {
                      n123 = Delete From Array(array=w478, index=w483) -> (array with subset deleted=w486:i32[])  [unwired: 1 in, 1 out]
                      n124 = Delete From Array(array=w477, index=w483) -> (array with subset deleted=w485:i32[])  [unwired: 1 in, 1 out]
                      n125 = Build Array (concatenate)(w486, w485) -> (w484:i32[])
                      n126 = call "Open Close Valves.vi"("Valves to Close"=w484, "Current Valve State"=w479, "Debug Mode"=w480, "Reactor Name"=w476, "Reactor Selector"=w475, "Pump Valves"=w478, "System Queue"=w482, "JSON Queue"=w481) -> ()  [unwired: 12 in]
                    }
                    frame #1 {
                      n127 = property class="DigNum (strict)"(reference=w487) -> ("Value"=w488:i32)  [unwired: 1 in, 2 out]
                      n128 = Wait (ms)(milliseconds to wait=w488) -> ()  [unwired: 1 out]
                    }
                    frame #2 {
                      n129 = call "Open Close Valves.vi"("Valves to Open"=w496, "Current Valve State"=w494, "Debug Mode"=w495, "Reactor Name"=w490, "Reactor Selector"=w489, "Pump Valves"=w491, "System Queue"=w493, "JSON Queue"=w492) -> ()  [unwired: 12 in]
                    }
                    frame #3 {
                      n130 = Tick Count (ms)() -> (millisecond timer value=w500:u32)
                      n131 = property class="DigNum (strict)"(reference=w499, "Value"=w500) -> ()  [unwired: 1 in, 2 out]
                      n132 = property class="DigNum (strict)"(reference=w498, "Value"=w497) -> ()  [unwired: 1 in, 2 out]
                    }
                  }
                  n133 = call "LogMessage.vi"("Type"=enum16{"Locks", "Warning"}."Warning", "Reactor Name"=w442, "Log Entry"="Initiating \"N2 Overlap\"", "System JSON Queue"=w451, "ID Number"=w459, "System Queue"=w452) -> ()
                }
              }
            }
            frame "9-Wait N2Overlap" {
              n134 = property class="DigNum (strict)"(reference=w534) -> ("Value"=w537:i32)  [unwired: 1 in, 2 out]
              n135 = Tick Count (ms)() -> (millisecond timer value=w536:u32)
              n136 = Subtract(x=w536, y=w537) -> (x-y=w538:u32)
              n137 = Multiply(x=w533, y=1000) -> (x*y=w539:dbl)
              n138 = Less?(x=w538, y=w539) -> (x < y?=w535:bool)
              n139 = case shown="False" w535 {
                tunnel: [Valve_State_Machine."10-Init Pump Overlap" Valve_State_Machine."9-Wait N2Overlap"] -> w543
                tunnel: w532 -> [w548 _]
                tunnel: w531 -> [w552 _]
                tunnel: w530 -> [w550 _]
                tunnel: w529 -> [w551 _]
                tunnel: w528 -> [w549 _]
                tunnel: w527 -> [w558 _]
                tunnel: w526 -> [w557 _]
                tunnel: w525 -> [w556 _]
                tunnel: w524 -> [w555 _]
                tunnel: w523 -> [w554 _]
                tunnel: w522 -> [w546 _]
                tunnel: w521 -> [w544 _]
                frame False {
                  n140 = Greater?(x=w548, y=50) -> (0:w545:bool)
                  n141 = case shown="True" w545 {
                    tunnel: [w577 w580] -> w553
                    tunnel: w552 -> [w573 w581]
                    tunnel: w550 -> [w571 _]
                    tunnel: w551 -> [w570 w579]
                    tunnel: w549 -> [w565 _]
                    tunnel: w548 -> [w569 _]
                    frame True {
                      n142 = Quotient & Remainder(x=w569, y=10) -> (floor(x/y)=w568:i32)  [unwired: 1 out]
                      n143 = Subtract(x=w568, y=5) -> (x-y=w566:i32)
                      n144 = Multiply(x=w566, y=w565) -> (x*y=w564:i32)
                      n145 = call "Local to Global Valve Numbers.vi"("Reactor ID #"=w573, "List of Local Valves"=i32[] [1], "Valves Per Reactor"=w570) -> ("List of Global Valves"=w572:i32[])  [unwired: 2 in]
                      n146 = Multiply(x=w570, y=w571) -> (x*y=w576:i32)
                      n147 = Add(x=w576, y=w564) -> (x+y=w575:i32)
                      n148 = Increment(x=w575) -> (x+1=w578:i32)
                      n149 = Build Array (concatenate)(w572, w578) -> (w577:i32[])
                    }
                    frame False {
                      n150 = call "Local to Global Valve Numbers.vi"("Reactor ID #"=w581, "List of Local Valves"=i32[] [1, 2], "Valves Per Reactor"=w579) -> ("List of Global Valves"=w580:i32[])  [unwired: 2 in]
                    }
                  }
                  n151 = call "Convert Recipe Valve to Valve List.vi"("Valves on Shared Lines"=w549, "Valves Per Reactor"=w551, "Number of Reactors"=w550, "Reactor ID#"=w552, "Valve Number"=w548) -> ("Valve List"=w561:i32[])  [unwired: 10 in]
                  n152 = Build Array (concatenate)(w561, w553) -> (w560:i32[])
                  n153 = call "Open Close Valves.vi"("Valves to Open"=i32[] [], "Valves to Close"=w560, "Current Valve State"=w558, "Debug Mode"=w557, "Reactor Name"=w546, "Reactor Selector"=w544, "Pump Valves"=w554, "System Queue"=w556, "JSON Queue"=w555) -> ()  [unwired: 11 in]
                }
                frame True {
                  n154 = Wait (ms)(milliseconds to wait=u32 10 ("millisecond multiple")) -> ()  [unwired: 1 out]
                }
              }
            }
            frame "10-Init Pump Overlap" {
              n155 = Greater Than 0?(x=w605) -> (x > 0?=w607:bool)
              n156 = case shown="True" w607 {
                tunnel: [Valve_State_Machine."12-Release Pump Lock" Valve_State_Machine."11-Wait Pump Overlap"] -> w599
                tunnel: w605 -> [_ w621]
                tunnel: w606 -> [_ w622]
                tunnel: w603 -> [_ w640]
                tunnel: w601 -> [_ w624]
                tunnel: w602 -> [_ w627]
                tunnel: w604 -> [_ w636]
                tunnel: w597 -> [_ w628]
                tunnel: w596 -> [_ w620]
                tunnel: w595 -> [_ w619]
                tunnel: w594 -> [_ w618]
                tunnel: w593 -> [_ w616]
                tunnel: w592 -> [_ w617]
                tunnel: w591 -> [_ w615]
                tunnel: w590 -> [_ w611]
                tunnel: w589 -> [_ w614]
                tunnel: w588 -> [_ w613]
                tunnel: w587 -> [_ w612]
                tunnel: w586 -> [_ w610]
                tunnel: w585 -> [_ w609]
                frame False {
                }
                frame True {
                  # "Pump Open\nNitrogen Closed"
                  n157 = call "Local to Global Valve Numbers.vi"("Reactor ID #"=w624, "List of Local Valves"=i32[] [1], "Valves Per Reactor"=w619) -> ("List of Global Valves"=w631:i32[])  [unwired: 2 in]
                  n158 = call "Convert Recipe Valve to Valve List.vi"("Valves on Shared Lines"=w620, "Valves Per Reactor"=w619, "Number of Reactors"=w618, "Reactor ID#"=w624, "Valve Number"=w627) -> ("Valve List"=w635:i32[])  [unwired: 10 in]
                  n159 = Build Array (concatenate)(w635, w631) -> (w634:i32[])
                  n160 = Subtract(x=w640, y=1) -> (x-y=w643:i32)
                  n161 = Bundle(w643, 4) -> (w639:cluster{i32, i32})  [unwired: 1 in]
                  n162 = Decrement(x=w624) -> (x-1=w630:i32)
                  n163 = property class="Tbl (strict)"(reference=w636, "Cell BG Color"=u32 12123391, "Active Cell"=w639, "Cell BG Color"=u32 16318208) -> ()  [unwired: 1 in, 2 out]
                  n164 = Delete From Array(array=w616, index=w630) -> (array with subset deleted=w629:i32[])  [unwired: 1 in, 1 out]
                  n165 = Build Array (concatenate)(w629, w617) -> (w626:i32[])
                  n166 = stacked-sequence {
                    tunnel: w634 -> [_ _ w661 _]
                    tunnel: w628 -> [_ _ _ w664]
                    tunnel: w626 -> [w651 _ _ _]
                    tunnel: w622 -> [_ _ _ w663]
                    tunnel: w621 -> [_ _ _ w662]
                    tunnel: w616 -> [w650 _ w660 _]
                    tunnel: w615 -> [w649 _ w659 _]
                    tunnel: w611 -> [w648 _ w658 _]
                    tunnel: w614 -> [w647 _ w657 _]
                    tunnel: w613 -> [w646 _ w656 _]
                    tunnel: w612 -> [_ w653 _ _]
                    tunnel: w610 -> [w645 _ w655 _]
                    tunnel: w609 -> [w644 _ w654 _]
                    frame #0 {
                      n167 = call "Open Close Valves.vi"("Valves to Close"=w651, "Current Valve State"=w647, "Debug Mode"=w646, "Reactor Name"=w645, "Reactor Selector"=w644, "Pump Valves"=w650, "System Queue"=w649, "JSON Queue"=w648) -> ()  [unwired: 12 in]
                    }
                    frame #1 {
                      n168 = property class="DigNum (strict)"(reference=w653) -> ("Value"=w652:i32)  [unwired: 1 in, 2 out]
                      n169 = Wait (ms)(milliseconds to wait=w652) -> ()  [unwired: 1 out]
                    }
                    frame #2 {
                      n170 = call "Open Close Valves.vi"("Valves to Open"=w661, "Current Valve State"=w657, "Debug Mode"=w656, "Reactor Name"=w655, "Reactor Selector"=w654, "Pump Valves"=w660, "System Queue"=w659, "JSON Queue"=w658) -> ()  [unwired: 12 in]
                    }
                    frame #3 {
                      n171 = Tick Count (ms)() -> (millisecond timer value=w665:u32)
                      n172 = property class="DigNum (strict)"(reference=w664, "Value"=w665) -> ()  [unwired: 1 in, 2 out]
                      n173 = property class="DigNum (strict)"(reference=w663, "Value"=w662) -> ()  [unwired: 1 in, 2 out]
                    }
                  }
                  n174 = call "LogMessage.vi"("Type"=enum16{"Locks", "Warning"}."Warning", "Reactor Name"=w610, "Log Entry"="Initiating \"Pump Overlap\"", "System JSON Queue"=w611, "ID Number"=w624, "System Queue"=w615) -> ()
                }
              }
            }
            frame "11-Wait Pump Overlap" {
              n175 = property class="DigNum (strict)"(reference=w678) -> ("Value"=w682:i32)  [unwired: 1 in, 2 out]
              n176 = Tick Count (ms)() -> (millisecond timer value=w681:u32)
              n177 = Subtract(x=w681, y=w682) -> (x-y=w683:u32)
              n178 = Multiply(x=w679, y=1000) -> (x*y=w684:dbl)
              n179 = Less?(x=w683, y=w684) -> (x < y?=w680:bool)
              n180 = case shown="False" w680 {
                tunnel: [Valve_State_Machine."12-Release Pump Lock" Valve_State_Machine."11-Wait Pump Overlap"] -> w688
                tunnel: w677 -> [w700 _]
                tunnel: w676 -> [w699 _]
                tunnel: w675 -> [w698 _]
                tunnel: w674 -> [w697 _]
                tunnel: w673 -> [w696 _]
                tunnel: w672 -> [w695 _]
                tunnel: w671 -> [w694 _]
                tunnel: w670 -> [w693 _]
                tunnel: w669 -> [w692 _]
                tunnel: w668 -> [w691 _]
                tunnel: w667 -> [w690 _]
                tunnel: w666 -> [w689 _]
                frame False {
                  n181 = call "Local to Global Valve Numbers.vi"("Reactor ID #"=w700, "List of Local Valves"=i32[] [1], "Valves Per Reactor"=w694) -> ("List of Global Valves"=w704:i32[])  [unwired: 2 in]
                  n182 = call "Convert Recipe Valve to Valve List.vi"("Valves on Shared Lines"=w692, "Valves Per Reactor"=w694, "Number of Reactors"=w693, "Reactor ID#"=w700, "Valve Number"=w699) -> ("Valve List"=w705:i32[])  [unwired: 10 in]
                  n183 = Build Array (concatenate)(w705, w704) -> (w701:i32[])
                  n184 = call "Open Close Valves.vi"("Valves to Open"=i32[] [], "Valves to Close"=w701, "Current Valve State"=w698, "Debug Mode"=w697, "Reactor Name"=w690, "Reactor Selector"=w689, "Pump Valves"=w691, "System Queue"=w696, "JSON Queue"=w695) -> ()  [unwired: 11 in]
                }
                frame True {
                  n185 = Wait (ms)(milliseconds to wait=u32 10 ("millisecond multiple")) -> ()  [unwired: 1 out]
                }
              }
            }
            frame "12-Release Pump Lock" {
              n186 = call "Lockout.vi"("Locks"=w710, "ID"=w715, "Queue System"=w712, "Request Type"=enum16{"Lock", "Release", "Check"}."Release", "Request Array"=i32[] [0], "Reactor Name"=w709, "JSON Queue"=w711) -> ()  [unwired: 2 out]
              n187 = Wait (ms)(milliseconds to wait=u32 250) -> ()  [unwired: 1 out]
            }
            frame "13-Init Open Time" {
              n188 = Greater Than 0?(x=w740) -> (x > 0?=w741:bool)
              n189 = case shown="True" w741 {
                tunnel: [Valve_State_Machine."15-Release All Locks" Valve_State_Machine."14-Wait Open Time"] -> w734
                tunnel: w740 -> [_ w754]
                tunnel: w739 -> [_ w755]
                tunnel: w738 -> [_ w769]
                tunnel: w735 -> [_ w757]
                tunnel: w736 -> [_ w764]
                tunnel: w737 -> [_ w765]
                tunnel: w731 -> [_ w759]
                tunnel: w730 -> [_ w753]
                tunnel: w729 -> [_ w752]
                tunnel: w728 -> [_ w751]
                tunnel: w727 -> [_ w750]
                tunnel: w726 -> [_ w749]
                tunnel: w725 -> [_ w748]
                tunnel: w724 -> [_ w747]
                tunnel: w723 -> [_ w746]
                tunnel: w722 -> [_ w745]
                tunnel: w721 -> [_ w744]
                tunnel: w720 -> [_ w743]
                frame False {
                }
                frame True {
                  # "Pump Closed\nNitrogen Closed"
                  n190 = call "Convert Recipe Valve to Valve List.vi"("Valves on Shared Lines"=w746, "Valves Per Reactor"=w747, "Number of Reactors"=w748, "Reactor ID#"=w757, "Valve Number"=w764) -> ("Valve List"=w763:i32[])  [unwired: 10 in]
                  n191 = Subtract(x=w769, y=1) -> (x-y=w772:i32)
                  n192 = call "Local to Global Valve Numbers.vi"("Reactor ID #"=w757, "List of Local Valves"=i32[] [1, 2], "Valves Per Reactor"=w747) -> ("List of Global Valves"=w760:i32[])  [unwired: 2 in]
                  n193 = Bundle(w772, 5) -> (w768:cluster{i32, i32})  [unwired: 1 in]
                  n194 = call "LogMessage.vi"("Type"=enum16{"Locks", "Warning"}."Warning", "Reactor Name"=w744, "Log Entry"="Initiating \"Dose\"", "System JSON Queue"=w750, "ID Number"=w757, "System Queue"=w751) -> ()
                  n195 = property class="Tbl (strict)"(reference=w765, "Cell BG Color"=u32 12123391, "Active Cell"=w768, "Cell BG Color"=u32 16318208) -> ()  [unwired: 1 in, 2 out]
                  n196 = stacked-sequence {
                    tunnel: w752 -> [w780 _ w790 _]
                    tunnel: w763 -> [_ _ w788 _]
                    tunnel: w760 -> [w779 _ _ _]
                    tunnel: w745 -> [w778 _ w787 _]
                    tunnel: w751 -> [w777 _ w789 _]
                    tunnel: w759 -> [_ _ _ w793]
                    tunnel: w750 -> [w776 _ w786 _]
                    tunnel: w753 -> [w775 _ w785 _]
                    tunnel: w755 -> [_ _ _ w792]
                    tunnel: w754 -> [_ _ _ w791]
                    tunnel: w749 -> [_ w781 _ _]
                    tunnel: w744 -> [w774 _ w784 _]
                    tunnel: w743 -> [w773 _ w783 _]
                    frame #0 {
                      n197 = call "Open Close Valves.vi"("Valves to Close"=w779, "Current Valve State"=w780, "Debug Mode"=w775, "Reactor Name"=w774, "Reactor Selector"=w773, "Pump Valves"=w778, "System Queue"=w777, "JSON Queue"=w776) -> ()  [unwired: 12 in]
                    }
                    frame #1 {
                      n198 = property class="DigNum (strict)"(reference=w781) -> ("Value"=w782:i32)  [unwired: 1 in, 2 out]
                      n199 = Wait (ms)(milliseconds to wait=w782) -> ()  [unwired: 1 out]
                    }
                    frame #2 {
                      n200 = call "Open Close Valves.vi"("Valves to Open"=w788, "Current Valve State"=w790, "Debug Mode"=w785, "Reactor Name"=w784, "Reactor Selector"=w783, "Pump Valves"=w787, "System Queue"=w789, "JSON Queue"=w786) -> ()  [unwired: 12 in]
                    }
                    frame #3 {
                      n201 = Tick Count (ms)() -> (millisecond timer value=w794:u32)
                      n202 = property class="DigNum (strict)"(reference=w793, "Value"=w794) -> ()  [unwired: 1 in, 2 out]
                      n203 = property class="DigNum (strict)"(reference=w792, "Value"=w791) -> ()  [unwired: 1 in, 2 out]
                    }
                  }
                }
              }
            }
            frame "14-Wait Open Time" {
              n204 = property class="DigNum (strict)"(reference=w807) -> ("Value"=w811:i32)  [unwired: 1 in, 2 out]
              n205 = Tick Count (ms)() -> (millisecond timer value=w810:u32)
              n206 = Subtract(x=w810, y=w811) -> (x-y=w812:u32)
              n207 = Multiply(x=w808, y=1000) -> (x*y=w813:dbl)
              n208 = Less?(x=w812, y=w813) -> (x < y?=w809:bool)
              n209 = case shown="False" w809 {
                tunnel: [Valve_State_Machine."15-Release All Locks" Valve_State_Machine."14-Wait Open Time"] -> w817
                tunnel: w806 -> [w829 _]
                tunnel: w805 -> [w828 _]
                tunnel: w804 -> [w827 _]
                tunnel: w803 -> [w826 _]
                tunnel: w802 -> [w825 _]
                tunnel: w801 -> [w824 _]
                tunnel: w800 -> [w823 _]
                tunnel: w799 -> [w822 _]
                tunnel: w798 -> [w821 _]
                tunnel: w797 -> [w820 _]
                tunnel: w796 -> [w819 _]
                tunnel: w795 -> [w818 _]
                frame False {
                  n210 = call "Convert Recipe Valve to Valve List.vi"("Valves on Shared Lines"=w825, "Valves Per Reactor"=w827, "Number of Reactors"=w826, "Reactor ID#"=w829, "Valve Number"=w828) -> ("Valve List"=w830:i32[])  [unwired: 10 in]
                  n211 = call "Open Close Valves.vi"("Valves to Close"=w830, "Current Valve State"=w823, "Debug Mode"=w822, "Reactor Name"=w819, "Reactor Selector"=w818, "Pump Valves"=w824, "System Queue"=w821, "JSON Queue"=w820) -> ()  [unwired: 12 in]
                }
                frame True {
                  n212 = Wait (ms)(milliseconds to wait=u32 10 ("millisecond multiple")) -> ()  [unwired: 1 out]
                }
              }
            }
            frame "15-Release All Locks" {
              n213 = call "Lockout.vi"("Locks"=w837, "ID"=w840, "Queue System"=w836, "Request Type"=enum16{"Lock", "Release", "Check"}."Release", "Request Array"=i32[] [0, 1, 2], "Reactor Name"=w834, "JSON Queue"=w835) -> ()  [unwired: 2 out]
            }
            frame "16-Init Hold" {
              n214 = Greater Than 0?(x=w861) -> (x > 0?=w864:bool)
              n215 = case shown="True" w864 {
                tunnel: [Valve_State_Machine."18-Claim Pump Lock" Valve_State_Machine."17-Wait Hold"] -> w857
                tunnel: w861 -> [_ w876]
                tunnel: w862 -> [_ w877]
                tunnel: w859 -> [_ w893]
                tunnel: w858 -> [_ w879]
                tunnel: w863 -> [_ w888]
                tunnel: w860 -> [_ w889]
                tunnel: w854 -> [_ w881]
                tunnel: w853 -> [_ w875]
                tunnel: w852 -> [_ w874]
                tunnel: w851 -> [_ w873]
                tunnel: w850 -> [_ w872]
                tunnel: w849 -> [_ w871]
                tunnel: w848 -> [_ w869]
                tunnel: w847 -> [_ w868]
                tunnel: w846 -> [_ w870]
                tunnel: w845 -> [_ w867]
                tunnel: w844 -> [_ w866]
                frame False {
                }
                frame True {
                  # "All this is prob\nunnecessary.\nValves all should\nbe closed already."
                  # "Pump Closed\nNitrogen Closed"
                  n216 = call "Convert Recipe Valve to Valve List.vi"("Valves on Shared Lines"=w873, "Valves Per Reactor"=w875, "Number of Reactors"=w874, "Reactor ID#"=w879, "Valve Number"=w888) -> ("Valve List"=w884:i32[])  [unwired: 10 in]
                  n217 = Subtract(x=w893, y=1) -> (x-y=w896:i32)
                  n218 = call "Local to Global Valve Numbers.vi"("Reactor ID #"=w879, "List of Local Valves"=i32[] [1, 2], "Valves Per Reactor"=w875) -> ("List of Global Valves"=w885:i32[])  [unwired: 2 in]
                  n219 = Build Array (concatenate)(w885, w884) -> (w883:i32[])
                  n220 = Bundle(w896, 6) -> (w892:cluster{i32, i32})  [unwired: 1 in]
                  n221 = call "LogMessage.vi"("Type"=enum16{"Locks", "Warning"}."Warning", "Reactor Name"=w867, "Log Entry"="Initiating \"Soak Hold\"", "System JSON Queue"=w868, "ID Number"=w879, "System Queue"=w869) -> ()
                  n222 = property class="Tbl (strict)"(reference=w889, "Cell BG Color"=u32 12123391, "Active Cell"=w892, "Cell BG Color"=u32 16318208) -> ()  [unwired: 1 in, 2 out]
                  n223 = flat-sequence {
                    tunnel: w871 -> [w905]
                    tunnel: w883 -> [w904]
                    tunnel: i32[] [] ("Valves to Open") -> [w903]
                    tunnel: w872 -> [w902]
                    tunnel: w869 -> [w901]
                    tunnel: w868 -> [w900]
                    tunnel: w870 -> [w899]
                    tunnel: w867 -> [w898]
                    tunnel: w866 -> [w897]
                    tunnel: w881 -> [w908]
                    tunnel: w877 -> [w907]
                    tunnel: w876 -> [w906]
                    frame #0 {
                      n224 = call "Open Close Valves.vi"("Valves to Open"=w903, "Valves to Close"=w904, "Current Valve State"=w905, "Debug Mode"=w899, "Reactor Name"=w898, "Reactor Selector"=w897, "Pump Valves"=w902, "System Queue"=w901, "JSON Queue"=w900) -> ()  [unwired: 11 in]
                    }
                    frame #1 {
                      n225 = Tick Count (ms)() -> (millisecond timer value=w909:u32)
                      n226 = property class="DigNum (strict)"(reference=w908, "Value"=w909) -> ()  [unwired: 1 in, 2 out]
                      n227 = property class="DigNum (strict)"(reference=w907, "Value"=w906) -> ()  [unwired: 1 in, 2 out]
                    }
                  }
                }
              }
            }
            frame "17-Wait Hold" {
              n228 = property class="DigNum (strict)"(reference=w911) -> ("Value"=w914:i32)  [unwired: 1 in, 2 out]
              n229 = Tick Count (ms)() -> (millisecond timer value=w913:u32)
              n230 = Subtract(x=w913, y=w914) -> (x-y=w915:u32)
              n231 = Multiply(x=w910, y=1000) -> (x*y=w916:dbl)
              n232 = Less?(x=w915, y=w916) -> (x < y?=w912:bool)
              n233 = case shown="True" w912 {
                tunnel: [Valve_State_Machine."18-Claim Pump Lock" Valve_State_Machine."17-Wait Hold"] -> w920
                frame False {
                }
                frame True {
                  n234 = Wait (ms)(milliseconds to wait=u32 10 ("millisecond multiple")) -> ()  [unwired: 1 out]
                }
              }
            }
            frame "18-Claim Pump Lock" {
              n235 = call "Lockout.vi"("Locks"=w926, "ID"=w932, "Queue System"=w928, "Request Type"=enum16{"Lock", "Release", "Check"}."Lock", "Request Array"=i32[] [0], "Reactor Name"=w924, "JSON Queue"=w927) -> ("Response"=w929:bool)  [unwired: 1 out]
              n236 = case shown="True" w929 {
                tunnel: [Valve_State_Machine."18-Claim Pump Lock" Valve_State_Machine."19-Init Pump Purge"] -> w935
                tunnel: w925 -> [w937 _]
                frame False {
                  n237 = property class="DigNum (strict)"(reference=w937) -> ("Value"=w936:i32)  [unwired: 1 in, 2 out]
                  n238 = Wait (ms)(milliseconds to wait=w936) -> ()  [unwired: 1 out]
                }
                frame True {
                }
              }
            }
            frame "19-Init Pump Purge" {
              n239 = Greater Than 0?(x=w950) -> (x > 0?=w958:bool)
              n240 = case shown="True" w958 {
                tunnel: [Valve_State_Machine."21-Release Pump Lock" Valve_State_Machine."20-Wait Pump Purge"] -> w954
                tunnel: w959 -> [_ w972]
                tunnel: w956 -> [_ w988]
                tunnel: w955 -> [_ w974]
                tunnel: w957 -> [_ w984]
                tunnel: w951 -> [_ w976]
                tunnel: w950 -> [_ w971]
                tunnel: w949 -> [_ w970]
                tunnel: w948 -> [_ w969]
                tunnel: w947 -> [_ w968]
                tunnel: w946 -> [_ w967]
                tunnel: w945 -> [_ w966]
                tunnel: w944 -> [_ w965]
                tunnel: w943 -> [_ w964]
                tunnel: w942 -> [_ w963]
                tunnel: w941 -> [_ w962]
                tunnel: w940 -> [_ w961]
                frame False {
                  # "Why would you never have a post purge? Skip to regular purge, I guess."
                }
                frame True {
                  # "Pump Open\nNitrogen Open"
                  n241 = Decrement(x=w974) -> (x-1=w980:i32)
                  n242 = Delete From Array(array=w969, index=w980) -> (array with subset deleted=w978:i32[])  [unwired: 1 in, 1 out]
                  n243 = Delete From Array(array=w970, index=w980) -> (array with subset deleted=w979:i32[])  [unwired: 1 in, 1 out]
                  n244 = Subtract(x=w988, y=1) -> (x-y=w991:i32)
                  n245 = call "Local to Global Valve Numbers.vi"("Reactor ID #"=w974, "List of Local Valves"=i32[] [1, 2], "Valves Per Reactor"=w968) -> ("List of Global Valves"=w981:i32[])  [unwired: 2 in]
                  n246 = Build Array (concatenate)(w979, w978) -> (w977:i32[])
                  n247 = Bundle(w991, 7) -> (w987:cluster{i32, i32})  [unwired: 1 in]
                  n248 = property class="Tbl (strict)"(reference=w984, "Cell BG Color"=u32 12123391, "Active Cell"=w987, "Cell BG Color"=u32 4194090) -> ()  [unwired: 1 in, 2 out]
                  n249 = stacked-sequence {
                    tunnel: w967 -> [w999 _ w1009 _]
                    tunnel: w981 -> [_ _ w1008 _]
                    tunnel: w977 -> [w996 _ _ _]
                    tunnel: w970 -> [w997 _ w1007 _]
                    tunnel: w966 -> [w998 _ w1006 _]
                    tunnel: w976 -> [_ _ _ w1012]
                    tunnel: w965 -> [w995 _ w1005 _]
                    tunnel: w964 -> [w994 _ w1004 _]
                    tunnel: w972 -> [_ _ _ w1011]
                    tunnel: w971 -> [_ _ _ w1010]
                    tunnel: w963 -> [_ w1000 _ _]
                    tunnel: w962 -> [w993 _ w1003 _]
                    tunnel: w961 -> [w992 _ w1002 _]
                    frame #0 {
                      n250 = call "Open Close Valves.vi"("Valves to Close"=w996, "Current Valve State"=w999, "Debug Mode"=w994, "Reactor Name"=w993, "Reactor Selector"=w992, "Pump Valves"=w997, "System Queue"=w998, "JSON Queue"=w995) -> ()  [unwired: 12 in]
                    }
                    frame #1 {
                      n251 = property class="DigNum (strict)"(reference=w1000) -> ("Value"=w1001:i32)  [unwired: 1 in, 2 out]
                      n252 = Wait (ms)(milliseconds to wait=w1001) -> ()  [unwired: 1 out]
                    }
                    frame #2 {
                      n253 = call "Open Close Valves.vi"("Valves to Open"=w1008, "Current Valve State"=w1009, "Debug Mode"=w1004, "Reactor Name"=w1003, "Reactor Selector"=w1002, "Pump Valves"=w1007, "System Queue"=w1006, "JSON Queue"=w1005) -> ()  [unwired: 12 in]
                    }
                    frame #3 {
                      n254 = Tick Count (ms)() -> (millisecond timer value=w1013:u32)
                      n255 = property class="DigNum (strict)"(reference=w1012, "Value"=w1013) -> ()  [unwired: 1 in, 2 out]
                      n256 = property class="DigNum (strict)"(reference=w1011, "Value"=w1010) -> ()  [unwired: 1 in, 2 out]
                    }
                  }
                  n257 = call "LogMessage.vi"("Type"=enum16{"Locks", "Warning"}."Warning", "Reactor Name"=w962, "Log Entry"="Initiating \"Pre-Purge\"", "System JSON Queue"=w965, "ID Number"=w974, "System Queue"=w966) -> ()
                }
              }
            }
            frame "20-Wait Pump Purge" {
              n258 = property class="DigNum (strict)"(reference=w1015) -> ("Value"=w1018:i32)  [unwired: 1 in, 2 out]
              n259 = Tick Count (ms)() -> (millisecond timer value=w1017:u32)
              n260 = Subtract(x=w1017, y=w1018) -> (x-y=w1019:u32)
              n261 = Multiply(x=w1014, y=1000) -> (x*y=w1020:dbl)
              n262 = Less?(x=w1019, y=w1020) -> (x < y?=w1016:bool)
              n263 = case shown="True" w1016 {
                tunnel: [Valve_State_Machine."21-Release Pump Lock" Valve_State_Machine."20-Wait Pump Purge"] -> w1024
                frame False {
                }
                frame True {
                  n264 = Wait (ms)(milliseconds to wait=u32 10 ("millisecond multiple")) -> ()  [unwired: 1 out]
                }
              }
            }
            frame "21-Release Pump Lock" {
              n265 = call "Lockout.vi"("Locks"=w1031, "ID"=w1033, "Queue System"=w1030, "Request Type"=enum16{"Lock", "Release", "Check"}."Release", "Request Array"=i32[] [0], "Reactor Name"=w1028, "JSON Queue"=w1029) -> ()  [unwired: 2 out]
            }
            frame "22-Init Purge" {
              n266 = Greater Than 0?(x=w1049) -> (x > 0?=w1054:bool)
              n267 = case shown="True" w1054 {
                tunnel: [Valve_State_Machine."21-Release Pump Lock" Valve_State_Machine."23-Wait Purge"] -> w1048
                tunnel: w1049 -> [_ w1065]
                tunnel: w1053 -> [_ w1066]
                tunnel: w1051 -> [_ w1074]
                tunnel: w1050 -> [_ w1069]
                tunnel: w1052 -> [_ w1076]
                tunnel: [TRUE FALSE] -> w1047
                tunnel: w1046 -> [_ w1078]
                tunnel: w1045 -> [_ w1064]
                tunnel: w1044 -> [_ w1063]
                tunnel: w1043 -> [_ w1062]
                tunnel: w1042 -> [_ w1061]
                tunnel: w1041 -> [_ w1060]
                tunnel: w1040 -> [_ w1059]
                tunnel: w1039 -> [_ w1058]
                tunnel: w1038 -> [_ w1057]
                frame False {
                }
                frame True {
                  # "Need this in case jump straight to purge."
                  # "Pump Open\nNitrogen Open"
                  n268 = call "Local to Global Valve Numbers.vi"("Reactor ID #"=w1069, "List of Local Valves"=i32[] [1, 2], "Valves Per Reactor"=w1059) -> ("List of Global Valves"=w1081:i32[])  [unwired: 2 in]
                  n269 = call "LogMessage.vi"("Type"=enum16{"Locks", "Warning"}."Warning", "Reactor Name"=w1058, "Log Entry"="Initiating \"Purge\"", "System JSON Queue"=w1064, "ID Number"=w1069, "System Queue"=w1063) -> ()
                  n270 = Subtract(x=w1074, y=1) -> (x-y=w1072:i32)
                  n271 = Bundle(w1072, 8) -> (w1070:cluster{i32, i32})  [unwired: 1 in]
                  n272 = property class="Tbl (strict)"(reference=w1076, "Cell BG Color"=u32 12123391, "Active Cell"=w1070, "Cell BG Color"=u32 16318208) -> ()  [unwired: 1 in, 2 out]
                  n273 = flat-sequence {
                    tunnel: w1060 -> [w1092]
                    tunnel: w1081 -> [w1091]
                    tunnel: i32[] [] ("Valves to Close") -> [w1090]
                    tunnel: w1062 -> [w1089]
                    tunnel: w1063 -> [w1088]
                    tunnel: w1064 -> [w1087]
                    tunnel: w1061 -> [w1086]
                    tunnel: w1058 -> [w1085]
                    tunnel: w1057 -> [w1084]
                    tunnel: w1078 -> [w1095]
                    tunnel: w1066 -> [w1094]
                    tunnel: w1065 -> [w1093]
                    frame #0 {
                      n274 = call "Open Close Valves.vi"("Valves to Open"=w1091, "Valves to Close"=w1090, "Current Valve State"=w1092, "Debug Mode"=w1086, "Reactor Name"=w1085, "Reactor Selector"=w1084, "Pump Valves"=w1089, "System Queue"=w1088, "JSON Queue"=w1087) -> ()  [unwired: 11 in]
                    }
                    frame #1 {
                      n275 = Tick Count (ms)() -> (millisecond timer value=w1096:u32)
                      n276 = property class="DigNum (strict)"(reference=w1094, "Value"=w1093) -> ()  [unwired: 1 in, 2 out]
                      n277 = property class="DigNum (strict)"(reference=w1095, "Value"=w1096) -> ()  [unwired: 1 in, 2 out]
                    }
                  }
                }
              }
            }
            frame "23-Wait Purge" {
              n278 = property class="DigNum (strict)"(reference=w1102) -> ("Value"=w1106:i32)  [unwired: 1 in, 2 out]
              n279 = Tick Count (ms)() -> (millisecond timer value=w1105:u32)
              n280 = Subtract(x=w1105, y=w1106) -> (x-y=w1107:u32)
              n281 = Multiply(x=w1104, y=1000) -> (x*y=w1108:dbl)
              n282 = Less?(x=w1107, y=w1108) -> (x < y?=w1103:bool)
              n283 = case shown="True" w1103 {
                tunnel: [Valve_State_Machine."23-Wait Purge" w1139] -> w1113
                tunnel: [TRUE FALSE] -> w1114
                tunnel: [w1123 w1138] -> w1112
                tunnel: w1104 -> [w1123 w1137]
                tunnel: w1111 -> [w1119 w1136]
                tunnel: w1111 -> [_ w1135]
                tunnel: w1110 -> [w1121 _]
                tunnel: w1102 -> [_ w1134]
                tunnel: w1101 -> [_ w1133]
                tunnel: w1100 -> [_ w1129]
                tunnel: w1099 -> [w1117 w1128]
                tunnel: w1098 -> [w1116 w1127]
                tunnel: w1097 -> [w1115 w1126]
                frame False {
                  n284 = property class="Tbl (strict)"(reference=w1121, "Cell BG Color"=u32 12123391) -> ()  [unwired: 1 in, 2 out]
                  n285 = call "LogMessage.vi"("Type"=enum16{"Locks", "Warning"}."Warning", "Reactor Name"=w1115, "Log Entry"="Half-cycle Finished", "System JSON Queue"=w1116, "ID Number"=w1119, "System Queue"=w1117) -> ()
                }
                frame True {
                  n286 = call "Local to Global Valve Numbers.vi"("Reactor ID #"=w1136, "List of Local Valves"=i32[] [1], "Valves Per Reactor"=w1129) -> ("List of Global Valves"=w1144:i32[])  [unwired: 2 in]
                  n287 = Index Array(array=w1144, index=0) -> (element=w1142:i32)
                  n288 = property class="Arr (strict)"(reference=w1133) -> ("Value"=w1132:bool[])  [unwired: 1 in, 2 out]
                  n289 = Decrement(x=w1142) -> (x-1=w1141:i32)
                  n290 = Variant To Data(type=bool[] [], Variant=w1132) -> (data=w1131:bool[])  [unwired: 1 in, 1 out]
                  n291 = Index Array(array=w1131, index=w1141) -> (element=w1140:bool)
                  n292 = case shown="False" w1140 {
                    tunnel: [Valve_State_Machine."24-Check Purge Resume" Valve_State_Machine."23-Wait Purge"] -> w1139
                    tunnel: [w1154 w1164] -> w1138
                    tunnel: w1137 -> [w1159 w1164]
                    tunnel: w1135 -> [w1151 _]
                    tunnel: w1134 -> [w1155 _]
                    tunnel: w1128 -> [w1149 _]
                    tunnel: w1127 -> [w1148 _]
                    tunnel: w1126 -> [w1147 _]
                    frame False {
                      # "Pump Lock interupt:\nStop Countdown\nWait until lock is off to resume."
                      n293 = property class="DigNum (strict)"(reference=w1155) -> ("Value"=w1161:i32)  [unwired: 1 in, 2 out]
                      n294 = call "LogMessage.vi"("Type"=enum16{"Locks", "Warning"}."Warning", "Reactor Name"=w1147, "Log Entry"="Pump Lock Claimed. Wait to resume.", "System JSON Queue"=w1148, "ID Number"=w1151, "System Queue"=w1149) -> ()
                      n295 = Tick Count (ms)() -> (millisecond timer value=w1162:u32)
                      n296 = Subtract(x=w1162, y=w1161) -> (x-y=w1157:u32)
                      n297 = Multiply(x=w1159, y=1000) -> (x*y=w1158:dbl)
                      n298 = Subtract(x=w1158, y=w1157) -> (x-y=w1156:dbl)
                      n299 = Divide(x=w1156, y=1000.0) -> (x/y=w1154:dbl)
                    }
                    frame True {
                      n300 = Wait (ms)(milliseconds to wait=u32 250 ("millisecond multiple")) -> ()  [unwired: 1 out]
                    }
                  }
                }
              }
            }
            frame "24-Check Purge Resume" {
              n301 = call "Lockout.vi"("Locks"=w1171, "ID"=0, "Queue System"=w1169, "Request Type"=enum16{"Lock", "Release", "Check"}."Check", "Request Array"=i32[] [0], "Reactor Name"=w1167, "JSON Queue"=w1170) -> ("Response"=w1175:bool)  [unwired: 1 out]
              n302 = case shown="True" w1175 {
                tunnel: [Valve_State_Machine."24-Check Purge Resume" Valve_State_Machine."22-Init Purge"] -> w1179
                tunnel: w1177 -> [w1184 _]
                tunnel: w1176 -> [w1182 _]
                tunnel: w1168 -> [w1181 _]
                frame False {
                  # "Lock not cleared. Reset countdown and loop."
                  n303 = property class="DigNum (strict)"(reference=w1181) -> ("Value"=w1180:i32)  [unwired: 1 in, 2 out]
                  n304 = property class="DigNum (strict)"(reference=w1184, "Value"=w1182) -> ()  [unwired: 1 in, 2 out]
                  n305 = Wait (ms)(milliseconds to wait=w1180) -> ()  [unwired: 1 out]
                }
                frame True {
                  # "Lock cleared, resume"
                }
              }
            }
          }
          n306 = property class="Bool (strict)"(reference=w170) -> ("Value"=w169:bool)  [unwired: 1 in, 2 out]
          n307 = Not(x=w169) -> (.not. x?=w135:bool)
          n308 = property class="Bool (strict)"(reference=w136) -> ("Value"=w134:bool)  [unwired: 1 in, 2 out]
          n309 = Or(x=w134, y=w135) -> (x .or. y?=w137:bool)
          n310 = Or(x=w137, y=w151) -> (x .or. y?=w150:bool)
        }
        n311 = case shown="True" w110 {
          tunnel: w109 -> [_ w127]
          frame False {
          }
          frame True {
            n312 = property class="Tbl (strict)"(reference=w127, "Cell BG Color"=u32 12123391) -> ()  [unwired: 1 in, 2 out]
          }
        }
      }
    }
  }
